vi "Launch.vi"() -> ()   [LabVIEW 2019]
uses:
  Components/ViPER.lvlibp/1abvi3w/ProjectTemplates/Source/Core/ViPER/Components_Src/ViPER/ViPER.lvclass
panel:
  in  "Config XML":string="<?xml version=\"1.0\" encoding=\"UTF-8\" standalone=\"no\" ?>\n<Object>\n\n  <Name>Switch_Mgr</Name>\n\n  <Class>Switch_Manager</Class>\n\n  <Objects>\n    <Object>\n      <Name>Matrix_1</Name>\n      <Class>Switch_Keysight_34934A</Class>\n      <Config>\n        <NumElts>4</NumElts>\n        <Refnum>\n          <Name>VISA</Name>\n          <RefKind>VISA</RefKind>\n          <Val>USB0::0x0957::0x0507::MY56485422::INSTR</Val>\n</Refnum>\n        <I32>\n          <Name>Slot</Name>\n          <Val>1</Val>\n</I32>\n        <Array>\n          <Name>SwitchMap</Name>\n          <Dimsize>65</Dimsize>\n          <Cluster>\n            <Name>Alias</Name>\n            <NumElts>6</NumElts>\n            <String>\n              <Name>Name</Name>\n              <Val>Passive_Tests</Val>\n</String>\n            <Array>\n              <Name>Route</Name>\n              <Dimsize>0</Dimsize>\n              <String>\n                <Name>String</Name>\n                <Val/>\n</String>\n</Array>\n            <Array>\n              <Name>UnRoute</Name>\n              <Dimsize>0</Dimsize>\n              <String>\n                <Name>String</Name>\n                <Val/>\n</String>\n</Array>\n            <String>\n              <Name>Description</Name>\n              <Val>Tests component values unpowered</Val>\n</String>\n            <String>\n              <Name>Group</Name>\n              <Val/>\n</String>\n            <Boolean>\n              <Name>IsGroup</Name>\n              <Val>1</Val>\n</Boolean>\n</Cluster>\n          <Cluster>\n            <Name>Alias</Name>\n            <NumElts>6</NumElts>\n            <String>\n              <Name>Name</Name>\n              <Val>Discharge_C108_C109</Val>\n</String>\n            <Array>\n              <Name>Route</Name>\n              <Dimsize>4</Dimsize>\n              <String>\n                <Name>String</Name>\n                <Val>M1H:1:6:1</Val>\n</String>\n              <String>\n                <Name>String</Name>\n                <Val>M1H:1:19:1</Val>\n</String>\n              <String>\n                <Name>String</Name>\n                <Val>M1L:1:6:1</Val>\n</String>\n              <String>\n                <Name>String</Name>\n                <Val>M1L:1:19:1</Val>\n</String>\n</Array>\n            <Array>\n              <Name>UnRoute</Name>\n              <Dimsize>4</Dimsize>\n              <String>\n                <Name>String</Name>\n                <Val>M1H:1:6:0</Val>\n</String>\n              <String>\n                <Name>String</Name>\n                <Val>M1H:1:19:0</Val>\n</String>\n              <String>\n                <Name>String</Name>\n                <Val>M1L:1:6:0</Val>\n</String>\n              <String>\n                <Name>String</Name>\n                <Val>M1L:1:19:0</Val>\n</String>\n</Array>\n            <String>\n              <Name>Description</Name>\n              <Val>Discharge the caps for 3 secs</Val>\n</String>\n            <String>\n              <Name>Group</Name>\n              <Val>Passive_Tests</Val>\n</String>\n            <Boolean>\n              <Name>IsGroup</Name>\n              <Val>0</Val>\n</Boolean>\n</Cluster>\n          <Cluster>\n            <Name>Alias</Name>\n            <NumElts>6</NumElts>\n            <String>\n              <Name>Name</Name>\n              <Val>Capacitors</Val>\n</String>\n            <Array>\n              <Name>Route</Name>\n              <Dimsize>0</Dimsize>\n              <String>\n                <Name>String</Name>\n                <Val/>\n</String>\n</Array>\n            <Array>\n              <Name>UnRoute</Name>\n              <Dimsize>0</Dimsize>\n              <String>\n                <Name>String</Name>\n                <Val/>\n</String>\n</Array>\n            <String>\n              <Name>Description</Name>\n              <Val>Tests Capacitor Values</Val>\n</String>\n            <String>\n              <Name>Group</Name>\n              <Val>Passive_Tests</Val>\n</String>\n            <Boolean>\n              <Name>IsGroup</Name>\n              <Val>1</Val>\n</Boolean>\n</Cluster>\n          <Cluster>\n            <Name>Alias</Name>\n            <NumElts>6</NumElts>\n            <String>\n              <Name>Name</Name>\n              <Val>Connect_LCR</Val>\n</String>\n            <Array>\n              <Name>Route</Name>\n              <Dimsize>4</Dimsize>\n              <String>\n                <Name>String</Name>\n                <Val>M1H:1:23:1</Val>\n</String>\n              <String>\n                <Name>String</Name>\n                <Val>M1H:2:24:1</Val>\n</String>\n              <String>\n                <Name>String</Name>\n                <Val>M1L:1:25:1</Val>\n</String>\n              <String>\n                <Name>String</Name>\n                <Val>M1L:2:26:1</Val>\n</String>\n</Array>\n            <Array>\n              <Name>UnRoute</Name>\n              <Dimsize>4</Dimsize>\n              <String>\n                <Name>String</Name>\n                <Val>M1H:1:23:0</Val>\n</String>\n              <String>\n                <Name>String</Name>\n                <Val>M1H:2:24:0</Val>\n</String>\n              <String>\n                <Name>String</Name>\n                <Val>M1L:1:25:0</Val>\n</String>\n              <String>\n                <Name>String</Name>\n                <Val>M1L:2:26:0</Val>\n</String>\n</Array>\n            <String>\n              <Name>Description</Name>\n              <Val>Connect the LCR to the Matrix</Val>\n</String>\n            <String>\n              <Name>Group</Name>\n              <Val>Capacitors</Val>\n</String>\n            <Boolean>\n              <Name>IsGroup</Name>\n              <Val>0</Val>\n</Boolean>\n</Cluster>\n          <Cluster>\n            <Name>Alias</Name>\n            <NumElts>6</NumElts>\n            <String>\n              <Name>Name</Name>\n              <Val>C108_C109</Val>\n</String>\n            <Array>\n              <Name>Route</Name>\n              <Dimsize>4</Dimsize>\n              <String>\n                <Name>String</Name>\n                <Val>M1H:1:6:1</Val>\n</String>\n              <String>\n                <Name>String</Name>\n                <Val>M1H:2:6:1</Val>\n</String>\n              <String>\n                <Name>String</Name>\n                <Val>M1L:1:6:1</Val>\n</String>\n              <String>\n                <Name>String</Name>\n                <Val>M1L:2:6:1</Val>\n</String>\n</Array>\n            <Array>\n              <Name>UnRoute</Name>\n              <Dimsize>4</Dimsize>\n              <String>\n                <Name>String</Name>\n                <Val>M1H:1:6:0</Val>\n</String>\n              <String>\n                <Name>String</Name>\n                <Val>M1H:2:6:0</Val>\n</String>\n              <String>\n                <Name>String</Name>\n                <Val>M1L:1:6:0</Val>\n</String>\n              <String>\n                <Name>String</Name>\n                <Val>M1L:2:6:0</Val>\n</String>\n</Array>\n            <String>\n              <Name>Description</Name>\n              <Val>C108 and C109 to LCR</Val>\n</String>\n            <String>\n              <Name>Group</Name>\n              <Val>Capacitors</Val>\n</String>\n            <Boolean>\n              <Name>IsGroup</Name>\n              <Val>0</Val>\n</Boolean>\n</Cluster>\n          <Cluster>\n            <Name>Alias</Name>\n            <NumElts>6</NumElts>\n            <String>\n              <Name>Name</Name>\n              <Val>C153</Val>\n</String>\n            <Array>\n              <Name>Route</Name>\n              <Dimsize>4</Dimsize>\n              <String>\n                <Name>String</Name>\n                <Val>M1H:1:7:1</Val>\n</String>\n              <String>\n                <Name>String</Name>\n                <Val>M1H:2:7:1</Val>\n</String>\n              <String>\n                <Name>String</Name>\n                <Val>M1L:1:5:1</Val>\n</String>\n              <String>\n                <Name>String</Name>\n                <Val>M1L:2:5:1</Val>\n</String>\n</Array>\n            <Array>\n              <Name>UnRoute</Name>\n              <Dimsize>4</Dimsize>\n              <String>\n                <Name>String</Name>\n                <Val>M1H:1:7:0</Val>\n</String>\n              <String>\n                <Name>String</Name>\n                <Val>M1H:2:7:0</Val>\n</String>\n              <String>\n                <Name>String</Name>\n                <Val>M1L:1:5:0</Val>\n</String>\n              <String>\n                <Name>String</Name>\n                <Val>M1L:2:5:0</Val>\n</String>\n</Array>\n            <String>\n              <Name>Description</Name>\n              <Val>C153 to LCR</Val>\n</String>\n            <String>\n              <Name>Group</Name>\n              <Val>Capacitors</Val>\n</String>\n            <Boolean>\n              <Name>IsGroup</Name>\n              <Val>0</Val>\n</Boolean>\n</Cluster>\n          <Cluster>\n            <Name>Alias</Name>\n            <NumElts>6</NumElts>\n            <String>\n              <Name>Name</Name>\n              <Val>C1300</Val>\n</String>\n            <Array>\n              <Name>Route</Name>\n              <Dimsize>4</Dimsize>\n              <String>\n                <Name>String</Name>\n                <Val>M1H:1:2:1</Val>\n</String>\n              <String>\n                <Name>String</Name>\n                <Val>M1H:2:2:1</Val>\n</String>\n              <String>\n                <Name>String</Name>\n                <Val>M1L:1:7:1</Val>\n</String>\n              <String>\n                <Name>String</Name>\n                <Val>M1L:2:7:1</Val>\n</String>\n</Array>\n            <Array>\n              <Name>UnRoute</Name>\n              <Dimsize>4</Dimsize>\n              <String>\n                <Name>String</Name>\n                <Val>M1H:1:2:0</Val>\n</String>\n              <String>\n                <Name>String</Name>\n                <Val>M1H:2:2:0</Val>\n</String>\n              <String>\n                <Name>String</Name>\n                <Val>M1L:1:7:0</Val>\n</String>\n              <String>\n                <Name>String</Name>\n                <Val>M1L:2:7:0</Val>\n</String>\n</Array>\n            <String>\n              <Name>Description</Name>\n              <Val>C1300 to LCR</Val>\n</String>\n            <String>\n              <Name>Group</Name>\n              <Val>Capacitors</Val>\n</String>\n            <Boolean>\n              <Name>IsGroup</Name>\n              <Val>0</Val>\n</Boolean>\n</Cluster>\n          <Cluster>\n            <Name>Alias</Name>\n            <NumElts>6</NumElts>\n            <String>\n              <Name>Name</Name>\n              <Val>C701</Val>\n</String>\n            <Array>\n              <Name>Route</Name>\n              <Dimsize>4</Dimsize>\n              <String>\n                <Name>String</Name>\n                <Val>M1H:1:8:1</Val>\n</String>\n              <String>\n                <Name>String</Name>\n                <Val>M1H:2:8:1</Val>\n</String>\n              <String>\n                <Name>String</Name>\n                <Val>M1L:1:2:1</Val>\n</String>\n              <String>\n                <Name>String</Name>\n                <Val>M1L:2:2:1</Val>\n</String>\n</Array>\n            <Array>\n              <Name>UnRoute</Name>\n              <Dimsize>4</Dimsize>\n              <String>\n                <Name>String</Name>\n                <Val>M1H:1:8:0</Val>\n</String>\n              <String>\n                <Name>String</Name>\n                <Val>M1H:2:8:0</Val>\n</String>\n              <String>\n                <Name>String</Name>\n                <Val>M1L:1:2:0</Val>\n</String>\n              <String>\n                <Name>String</Name>\n                <Val>M1L:2:2:0</Val>\n</String>\n</Array>\n            <String>\n              <Name>Description</Name>\n              <Val>C701 to LCR</Val>\n</String>\n            <String>\n              <Name>Group</Name>\n              <Val>Capacitors</Val>\n</String>\n            <Boolean>\n              <Name>IsGroup</Name>\n              <Val>0</Val>\n</Boolean>\n</Cluster>\n          <Cluster>\n            <Name>Alias</Name>\n            <NumElts>6</NumElts>\n            <String>\n              <Name>Name</Name>\n              <Val>C1202</Val>\n</String>\n            <Array>\n              <Name>Route</Name>\n              <Dimsize>4</Dimsize>\n              <String>\n                <Name>String</Name>\n                <Val>M1H:1:2:1</Val>\n</String>\n              <String>\n                <Name>String</Name>\n                <Val>M1H:2:2:1</Val>\n</String>\n              <String>\n                <Name>String</Name>\n                <Val>M1L:1:8:1</Val>\n</String>\n              <String>\n                <Name>String</Name>\n                <Val>M1L:2:8:1</Val>\n</String>\n</Array>\n            <Array>\n              <Name>UnRoute</Name>\n              <Dimsize>4</Dimsize>\n              <String>\n                <Name>String</Name>\n                <Val>M1H:1:2:0</Val>\n</String>\n              <String>\n                <Name>String</Name>\n                <Val>M1H:2:2:0</Val>\n</String>\n              <String>\n                <Name>String</Name>\n                <Val>M1L:1:8:0</Val>\n</String>\n              <String>\n                <Name>String</Name>\n                <Val>M1L:2:8:0</Val>\n</String>\n</Array>\n            <String>\n              <Name>Description</Name>\n              <Val>C1202 to LCR</Val>\n</String>\n            <String>\n              <Name>Group</Name>\n              <Val>Capacitors</Val>\n</String>\n            <Boolean>\n              <Name>IsGroup</Name>\n              <Val>0</Val>\n</Boolean>\n</Cluster>\n          <Cluster>\n            <Name>Alias</Name>\n            <NumElts>6</NumElts>\n            <String>\n              <Name>Name</Name>\n              <Val>C1204</Val>\n</String>\n            <Array>\n              <Name>Route</Name>\n              <Dimsize>4</Dimsize>\n              <String>\n                <Name>String</Name>\n                <Val>M1H:1:9:1</Val>\n</String>\n              <String>\n                <Name>String</Name>\n                <Val>M1H:2:9:1</Val>\n</String>\n              <String>\n                <Name>String</Name>\n                <Val>M1L:1:2:1</Val>\n</String>\n              <String>\n                <Name>String</Name>\n                <Val>M1L:2:2:1</Val>\n</String>\n</Array>\n            <Array>\n              <Name>UnRoute</Name>\n              <Dimsize>4</Dimsize>\n              <String>\n                <Name>String</Name>\n                <Val>M1H:1:9:0</Val>\n</String>\n              <String>\n                <Name>String</Name>\n                <Val>M1H:2:9:0</Val>\n</String>\n              <String>\n                <Name>String</Name>\n                <Val>M1L:1:2:0</Val>\n</String>\n              <String>\n                <Name>String</Name>\n                <Val>M1L:2:2:0</Val>\n</String>\n</Array>\n            <String>\n              <Name>Description</Name>\n              <Val>C1204 to LCR</Val>\n</String>\n            <String>\n              <Name>Group</Name>\n              <Val>Capacitors</Val>\n</String>\n            <Boolean>\n              <Name>IsGroup</Name>\n              <Val>0</Val>\n</Boolean>\n</Cluster>\n          <Cluster>\n            <Name>Alias</Name>\n            <NumElts>6</NumElts>\n            <String>\n              <Name>Name</Name>\n              <Val>C1200</Val>\n</String>\n            <Array>\n              <Name>Route</Name>\n              <Dimsize>4</Dimsize>\n              <String>\n                <Name>String</Name>\n                <Val>M1H:1:2:1</Val>\n</String>\n              <String>\n                <Name>String</Name>\n                <Val>M1H:2:2:1</Val>\n</String>\n              <String>\n                <Name>String</Name>\n                <Val>M1L:1:9:1</Val>\n</String>\n              <String>\n                <Name>String</Name>\n                <Val>M1L:2:9:1</Val>\n</String>\n</Array>\n            <Array>\n              <Name>UnRoute</Name>\n              <Dimsize>4</Dimsize>\n              <String>\n                <Name>String</Name>\n                <Val>M1H:1:2:0</Val>\n</String>\n              <String>\n                <Name>String</Name>\n                <Val>M1H:2:2:0</Val>\n</String>\n              <String>\n                <Name>String</Name>\n                <Val>M1L:1:9:0</Val>\n</String>\n              <String>\n                <Name>String</Name>\n                <Val>M1L:2:9:0</Val>\n</String>\n</Array>\n            <String>\n              <Name>Description</Name>\n              <Val>C1200 to LCR</Val>\n</String>\n            <String>\n              <Name>Group</Name>\n              <Val>Capacitors</Val>\n</String>\n            <Boolean>\n              <Name>IsGroup</Name>\n              <Val>0</Val>\n</Boolean>\n</Cluster>\n          <Cluster>\n            <Name>Alias</Name>\n            <NumElts>6</NumElts>\n            <String>\n              <Name>Name</Name>\n              <Val>Resistors</Val>\n</String>\n            <Array>\n              <Name>Route</Name>\n              <Dimsize>0</Dimsize>\n              <String>\n                <Name>String</Name>\n                <Val/>\n</String>\n</Array>\n            <Array>\n              <Name>UnRoute</Name>\n              <Dimsize>0</Dimsize>\n              <String>\n                <Name>String</Name>\n                <Val/>\n</String>\n</Array>\n            <String>\n              <Name>Description</Name>\n              <Val>Connect resistances to the DMM</Val>\n</String>\n            <String>\n              <Name>Group</Name>\n              <Val>Passive_Tests</Val>\n</String>\n            <Boolean>\n              <Name>IsGroup</Name>\n              <Val>1</Val>\n</Boolean>\n</Cluster>\n          <Cluster>\n            <Name>Alias</Name>\n            <NumElts>6</NumElts>\n            <String>\n              <Name>Name</Name>\n              <Val>24V_to_Gnd</Val>\n</String>\n            <Array>\n              <Name>Route</Name>\n              <Dimsize>0</Dimsize>\n              <String>\n                <Name>String</Name>\n                <Val/>\n</String>\n</Array>\n            <Array>\n              <Name>UnRoute</Name>\n              <Dimsize>0</Dimsize>\n              <String>\n                <Name>String</Name>\n                <Val/>\n</String>\n</Array>\n            <String>\n              <Name>Description</Name>\n              <Val>Ensure supply is not short circuit</Val>\n</String>\n            <String>\n              <Name>Group</Name>\n              <Val>Resistors</Val>\n</String>\n            <Boolean>\n              <Name>IsGroup</Name>\n              <Val>0</Val>\n</Boolean>\n</Cluster>\n          <Cluster>\n            <Name>Alias</Name>\n            <NumElts>6</NumElts>\n            <String>\n              <Name>Name</Name>\n              <Val>R121</Val>\n</String>\n            <Array>\n              <Name>Route</Name>\n              <Dimsize>4</Dimsize>\n              <String>\n                <Name>String</Name>\n                <Val>M1H:1:3:1</Val>\n</String>\n              <String>\n                <Name>String</Name>\n                <Val>M1H:2:3:1</Val>\n</String>\n              <String>\n                <Name>String</Name>\n                <Val>M1H:3:5:1</Val>\n</String>\n              <String>\n                <Name>String</Name>\n                <Val>M1H:4:5:1</Val>\n</String>\n</Array>\n            <Array>\n              <Name>UnRoute</Name>\n              <Dimsize>4</Dimsize>\n              <String>\n                <Name>String</Name>\n                <Val>M1H:1:3:0</Val>\n</String>\n              <String>\n                <Name>String</Name>\n                <Val>M1H:2:3:0</Val>\n</String>\n              <String>\n                <Name>String</Name>\n                <Val>M1H:3:5:0</Val>\n</String>\n              <String>\n                <Name>String</Name>\n                <Val>M1H:4:5:0</Val>\n</String>\n</Array>\n            <String>\n              <Name>Description</Name>\n              <Val>R121 to DMM</Val>\n</String>\n            <String>\n              <Name>Group</Name>\n              <Val>Resistors</Val>\n</String>\n            <Boolean>\n              <Name>IsGroup</Name>\n              <Val>0</Val>\n</Boolean>\n</Cluster>\n          <Cluster>\n            <Name>Alias</Name>\n            <NumElts>6</NumElts>\n            <String>\n              <Name>Name</Name>\n              <Val>LUG</Val>\n</String>\n            <Array>\n              <Name>Route</Name>\n              <Dimsize>4</Dimsize>\n              <String>\n                <Name>String</Name>\n                <Val>M1H:1:10:1</Val>\n</String>\n              <String>\n                <Name>String</Name>\n                <Val>M1H:2:10:1</Val>\n</String>\n              <String>\n                <Name>String</Name>\n                <Val>M1H:3:2:1</Val>\n</String>\n              <String>\n                <Name>String</Name>\n                <Val>M1H:4:2:1</Val>\n</String>\n</Array>\n            <Array>\n              <Name>UnRoute</Name>\n              <Dimsize>4</Dimsize>\n              <String>\n                <Name>String</Name>\n                <Val>M1H:1:10:0</Val>\n</String>\n              <String>\n                <Name>String</Name>\n                <Val>M1H:2:10:0</Val>\n</String>\n              <String>\n                <Name>String</Name>\n                <Val>M1H:3:2:0</Val>\n</String>\n              <String>\n                <Name>String</Name>\n                <Val>M1H:4:2:0</Val>\n</String>\n</Array>\n            <String>\n              <Name>Description</Name>\n              <Val>LUG to DMM</Val>\n</String>\n            <String>\n              <Name>Group</Name>\n              <Val>Resistors</Val>\n</String>\n            <Boolean>\n              <Name>IsGroup</Name>\n              <Val>0</Val>\n</Boolean>\n</Cluster>\n          <Cluster>\n            <Name>Alias</Name>\n            <NumElts>6</NumElts>\n            <String>\n              <Name>Name</Name>\n              <Val>R304</Val>\n</String>\n            <Array>\n              <Name>Route</Name>\n              <Dimsize>4</Dimsize>\n              <String>\n                <Name>String</Name>\n                <Val>M1L:1:10:1</Val>\n</String>\n              <String>\n                <Name>String</Name>\n                <Val>M1L:2:10:1</Val>\n</String>\n              <String>\n                <Name>String</Name>\n                <Val>M1L:3:2:1</Val>\n</String>\n              <String>\n                <Name>String</Name>\n                <Val>M1L:4:2:1</Val>\n</String>\n</Array>\n            <Array>\n              <Name>UnRoute</Name>\n              <Dimsize>4</Dimsize>\n              <String>\n                <Name>String</Name>\n                <Val>M1L:1:10:0</Val>\n</String>\n              <String>\n                <Name>String</Name>\n                <Val>M1L:2:10:0</Val>\n</String>\n              <String>\n                <Name>String</Name>\n                <Val>M1L:3:2:0</Val>\n</String>\n              <String>\n                <Name>String</Name>\n                <Val>M1L:4:2:0</Val>\n</String>\n</Array>\n            <String>\n              <Name>Description</Name>\n              <Val>R304 to DMM</Val>\n</String>\n            <String>\n              <Name>Group</Name>\n              <Val>Resistors</Val>\n</String>\n            <Boolean>\n              <Name>IsGroup</Name>\n              <Val>0</Val>\n</Boolean>\n</Cluster>\n          <Cluster>\n            <Name>Alias</Name>\n            <NumElts>6</NumElts>\n            <String>\n              <Name>Name</Name>\n              <Val>R203</Val>\n</String>\n            <Array>\n              <Name>Route</Name>\n              <Dimsize>4</Dimsize>\n              <String>\n                <Name>String</Name>\n                <Val>M1H:1:11:1</Val>\n</String>\n              <String>\n                <Name>String</Name>\n                <Val>M1H:2:11:1</Val>\n</String>\n              <String>\n                <Name>String</Name>\n                <Val>M1L:3:11:1</Val>\n</String>\n              <String>\n                <Name>String</Name>\n                <Val>M1L:4:11:1</Val>\n</String>\n</Array>\n            <Array>\n              <Name>UnRoute</Name>\n              <Dimsize>4</Dimsize>\n              <String>\n                <Name>String</Name>\n                <Val>M1H:1:11:0</Val>\n</String>\n              <String>\n                <Name>String</Name>\n                <Val>M1H:2:11:0</Val>\n</String>\n              <String>\n                <Name>String</Name>\n                <Val>M1L:3:11:0</Val>\n</String>\n              <String>\n                <Name>String</Name>\n                <Val>M1L:4:11:0</Val>\n</String>\n</Array>\n            <String>\n              <Name>Description</Name>\n              <Val>R203 to DMM</Val>\n</String>\n            <String>\n              <Name>Group</Name>\n              <Val>Resistors</Val>\n</String>\n            <Boolean>\n              <Name>IsGroup</Name>\n              <Val>0</Val>\n</Boolean>\n</Cluster>\n          <Cluster>\n            <Name>Alias</Name>\n            <NumElts>6</NumElts>\n            <String>\n              <Name>Name</Name>\n              <Val>R207</Val>\n</String>\n            <Array>\n              <Name>Route</Name>\n              <Dimsize>4</Dimsize>\n              <String>\n                <Name>String</Name>\n                <Val>M1H:1:16:1</Val>\n</String>\n              <String>\n                <Name>String</Name>\n                <Val>M1H:2:16:1</Val>\n</String>\n              <String>\n                <Name>String</Name>\n                <Val>M1L:3:15:1</Val>\n</String>\n              <String>\n                <Name>String</Name>\n                <Val>M1L:4:15:1</Val>\n</String>\n</Array>\n            <Array>\n              <Name>UnRoute</Name>\n              <Dimsize>4</Dimsize>\n              <String>\n                <Name>String</Name>\n                <Val>M1H:1:16:0</Val>\n</String>\n              <String>\n                <Name>String</Name>\n                <Val>M1H:2:16:0</Val>\n</String>\n              <String>\n                <Name>String</Name>\n                <Val>M1L:3:15:0</Val>\n</String>\n              <String>\n                <Name>String</Name>\n                <Val>M1L:4:15:0</Val>\n</String>\n</Array>\n            <String>\n              <Name>Description</Name>\n              <Val>R207 to DMM</Val>\n</String>\n            <String>\n              <Name>Group</Name>\n              <Val>Resistors</Val>\n</String>\n            <Boolean>\n              <Name>IsGroup</Name>\n              <Val>0</Val>\n</Boolean>\n</Cluster>\n          <Cluster>\n            <Name>Alias</Name>\n            <NumElts>6</NumElts>\n            <String>\n              <Name>Name</Name>\n              <Val>R200</Val>\n</String>\n            <Array>\n              <Name>Route</Name>\n              <Dimsize>4</Dimsize>\n              <String>\n                <Name>String</Name>\n                <Val>M1H:1:3:1</Val>\n</String>\n              <String>\n                <Name>String</Name>\n                <Val>M1H:2:3:1</Val>\n</String>\n              <String>\n                <Name>String</Name>\n                <Val>M1L:3:16:1</Val>\n</String>\n              <String>\n                <Name>String</Name>\n                <Val>M1L:4:16:1</Val>\n</String>\n</Array>\n            <Array>\n              <Name>UnRoute</Name>\n              <Dimsize>4</Dimsize>\n              <String>\n                <Name>String</Name>\n                <Val>M1H:1:3:0</Val>\n</String>\n              <String>\n                <Name>String</Name>\n                <Val>M1H:2:3:0</Val>\n</String>\n              <String>\n                <Name>String</Name>\n                <Val>M1L:3:16:0</Val>\n</String>\n              <String>\n                <Name>String</Name>\n                <Val>M1L:4:16:0</Val>\n</String>\n</Array>\n            <String>\n              <Name>Description</Name>\n              <Val>R200 to DMM</Val>\n</String>\n            <String>\n              <Name>Group</Name>\n              <Val>Resistors</Val>\n</String>\n            <Boolean>\n              <Name>IsGroup</Name>\n              <Val>0</Val>\n</Boolean>\n</Cluster>\n          <Cluster>\n            <Name>Alias</Name>\n            <NumElts>6</NumElts>\n            <String>\n              <Name>Name</Name>\n              <Val>R201</Val>\n</String>\n            <Array>\n              <Name>Route</Name>\n              <Dimsize>4</Dimsize>\n              <String>\n                <Name>String</Name>\n                <Val>M1H:1:3:1</Val>\n</String>\n              <String>\n                <Name>String</Name>\n                <Val>M1H:2:3:1</Val>\n</String>\n              <String>\n                <Name>String</Name>\n                <Val>M1H:3:17:1</Val>\n</String>\n              <String>\n                <Name>String</Name>\n                <Val>M1H:4:17:1</Val>\n</String>\n</Array>\n            <Array>\n              <Name>UnRoute</Name>\n              <Dimsize>4</Dimsize>\n              <String>\n                <Name>String</Name>\n                <Val>M1H:1:3:0</Val>\n</String>\n              <String>\n                <Name>String</Name>\n                <Val>M1H:2:3:0</Val>\n</String>\n              <String>\n                <Name>String</Name>\n                <Val>M1H:3:17:0</Val>\n</String>\n              <String>\n                <Name>String</Name>\n                <Val>M1H:4:17:0</Val>\n</String>\n</Array>\n            <String>\n              <Name>Description</Name>\n              <Val>R201 to DMM</Val>\n</String>\n            <String>\n              <Name>Group</Name>\n              <Val>Resistors</Val>\n</String>\n            <Boolean>\n              <Name>IsGroup</Name>\n              <Val>0</Val>\n</Boolean>\n</Cluster>\n          <Cluster>\n            <Name>Alias</Name>\n            <NumElts>6</NumElts>\n            <String>\n              <Name>Name</Name>\n              <Val>R215</Val>\n</String>\n            <Array>\n              <Name>Route</Name>\n              <Dimsize>4</Dimsize>\n              <String>\n                <Name>String</Name>\n                <Val>M1L:1:12:1</Val>\n</String>\n              <String>\n                <Name>String</Name>\n                <Val>M1L:2:12:1</Val>\n</String>\n              <String>\n                <Name>String</Name>\n                <Val>M1L:3:2:1</Val>\n</String>\n              <String>\n                <Name>String</Name>\n                <Val>M1L:4:2:1</Val>\n</String>\n</Array>\n            <Array>\n              <Name>UnRoute</Name>\n              <Dimsize>4</Dimsize>\n              <String>\n                <Name>String</Name>\n                <Val>M1L:1:12:0</Val>\n</String>\n              <String>\n                <Name>String</Name>\n                <Val>M1L:2:12:0</Val>\n</String>\n              <String>\n                <Name>String</Name>\n                <Val>M1L:3:2:0</Val>\n</String>\n              <String>\n                <Name>String</Name>\n                <Val>M1L:4:2:0</Val>\n</String>\n</Array>\n            <String>\n              <Name>Description</Name>\n              <Val>R215 to DMM</Val>\n</String>\n            <String>\n              <Name>Group</Name>\n              <Val>Resistors</Val>\n</String>\n            <Boolean>\n              <Name>IsGroup</Name>\n              <Val>0</Val>\n</Boolean>\n</Cluster>\n          <Cluster>\n            <Name>Alias</Name>\n            <NumElts>6</NumElts>\n            <String>\n              <Name>Name</Name>\n              <Val>R214</Val>\n</String>\n            <Array>\n              <Name>Route</Name>\n              <Dimsize>4</Dimsize>\n              <String>\n                <Name>String</Name>\n                <Val>M1H:1:2:1</Val>\n</String>\n              <String>\n                <Name>String</Name>\n                <Val>M1H:2:2:1</Val>\n</String>\n              <String>\n                <Name>String</Name>\n                <Val>M1L:3:12:1</Val>\n</String>\n              <String>\n                <Name>String</Name>\n                <Val>M1L:4:12:1</Val>\n</String>\n</Array>\n            <Array>\n              <Name>UnRoute</Name>\n              <Dimsize>4</Dimsize>\n              <String>\n                <Name>String</Name>\n                <Val>M1H:1:2:0</Val>\n</String>\n              <String>\n                <Name>String</Name>\n                <Val>M1H:2:2:0</Val>\n</String>\n              <String>\n                <Name>String</Name>\n                <Val>M1L:3:12:0</Val>\n</String>\n              <String>\n                <Name>String</Name>\n                <Val>M1L:4:12:0</Val>\n</String>\n</Array>\n            <String>\n              <Name>Description</Name>\n              <Val>R214 to DMM</Val>\n</String>\n            <String>\n              <Name>Group</Name>\n              <Val>Resistors</Val>\n</String>\n            <Boolean>\n              <Name>IsGroup</Name>\n              <Val>0</Val>\n</Boolean>\n</Cluster>\n          <Cluster>\n            <Name>Alias</Name>\n            <NumElts>6</NumElts>\n            <String>\n              <Name>Name</Name>\n              <Val>R412</Val>\n</String>\n            <Array>\n              <Name>Route</Name>\n              <Dimsize>4</Dimsize>\n              <String>\n                <Name>String</Name>\n                <Val>M1L:1:3:1</Val>\n</String>\n              <String>\n                <Name>String</Name>\n                <Val>M1L:2:3:1</Val>\n</String>\n              <String>\n                <Name>String</Name>\n                <Val>M1L:3:17:1</Val>\n</String>\n              <String>\n                <Name>String</Name>\n                <Val>M1L:4:17:1</Val>\n</String>\n</Array>\n            <Array>\n              <Name>UnRoute</Name>\n              <Dimsize>4</Dimsize>\n              <String>\n                <Name>String</Name>\n                <Val>M1L:1:3:0</Val>\n</String>\n              <String>\n                <Name>String</Name>\n                <Val>M1L:2:3:0</Val>\n</String>\n              <String>\n                <Name>String</Name>\n                <Val>M1L:3:17:0</Val>\n</String>\n              <String>\n                <Name>String</Name>\n                <Val>M1L:4:17:0</Val>\n</String>\n</Array>\n            <String>\n              <Name>Description</Name>\n              <Val>R412 to DMM</Val>\n</String>\n            <String>\n              <Name>Group</Name>\n              <Val>Resistors</Val>\n</String>\n            <Boolean>\n              <Name>IsGroup</Name>\n              <Val>0</Val>\n</Boolean>\n</Cluster>\n          <Cluster>\n            <Name>Alias</Name>\n            <NumElts>6</NumElts>\n            <String>\n              <Name>Name</Name>\n              <Val>R413</Val>\n</String>\n            <Array>\n              <Name>Route</Name>\n              <Dimsize>4</Dimsize>\n              <String>\n                <Name>String</Name>\n                <Val>M1H:1:13:1</Val>\n</String>\n              <String>\n                <Name>String</Name>\n                <Val>M1H:2:13:1</Val>\n</String>\n              <String>\n                <Name>String</Name>\n                <Val>M1H:3:2:1</Val>\n</String>\n              <String>\n                <Name>String</Name>\n                <Val>M1H:4:2:1</Val>\n</String>\n</Array>\n            <Array>\n              <Name>UnRoute</Name>\n              <Dimsize>4</Dimsize>\n              <String>\n                <Name>String</Name>\n                <Val>M1H:1:13:0</Val>\n</String>\n              <String>\n                <Name>String</Name>\n                <Val>M1H:2:13:0</Val>\n</String>\n              <String>\n                <Name>String</Name>\n                <Val>M1H:3:2:0</Val>\n</String>\n              <String>\n                <Name>String</Name>\n                <Val>M1H:4:2:0</Val>\n</String>\n</Array>\n            <String>\n              <Name>Description</Name>\n              <Val>R413 to DMM</Val>\n</String>\n            <String>\n              <Name>Group</Name>\n              <Val>Resistors</Val>\n</String>\n            <Boolean>\n              <Name>IsGroup</Name>\n              <Val>0</Val>\n</Boolean>\n</Cluster>\n          <Cluster>\n            <Name>Alias</Name>\n            <NumElts>6</NumElts>\n            <String>\n              <Name>Name</Name>\n              <Val>R416</Val>\n</String>\n            <Array>\n              <Name>Route</Name>\n              <Dimsize>4</Dimsize>\n              <String>\n                <Name>String</Name>\n                <Val>M1L:1:13:1</Val>\n</String>\n              <String>\n                <Name>String</Name>\n                <Val>M1L:2:13:1</Val>\n</String>\n              <String>\n                <Name>String</Name>\n                <Val>M1L:3:2:1</Val>\n</String>\n              <String>\n                <Name>String</Name>\n                <Val>M1L:4:2:1</Val>\n</String>\n</Array>\n            <Array>\n              <Name>UnRoute</Name>\n              <Dimsize>4</Dimsize>\n              <String>\n                <Name>String</Name>\n                <Val>M1L:1:13:0</Val>\n</String>\n              <String>\n                <Name>String</Name>\n                <Val>M1L:2:13:0</Val>\n</String>\n              <String>\n                <Name>String</Name>\n                <Val>M1L:3:2:0</Val>\n</String>\n              <String>\n                <Name>String</Name>\n                <Val>M1L:4:2:0</Val>\n</String>\n</Array>\n            <String>\n              <Name>Description</Name>\n              <Val>R416 to DMM</Val>\n</String>\n            <String>\n              <Name>Group</Name>\n              <Val>Resistors</Val>\n</String>\n            <Boolean>\n              <Name>IsGroup</Name>\n              <Val>0</Val>\n</Boolean>\n</Cluster>\n          <Cluster>\n            <Name>Alias</Name>\n            <NumElts>6</NumElts>\n            <String>\n              <Name>Name</Name>\n              <Val>SP500</Val>\n</String>\n            <Array>\n              <Name>Route</Name>\n              <Dimsize>4</Dimsize>\n              <String>\n                <Name>String</Name>\n                <Val>M1H:1:14:1</Val>\n</String>\n              <String>\n                <Name>String</Name>\n                <Val>M1H:2:14:1</Val>\n</String>\n              <String>\n                <Name>String</Name>\n                <Val>M1H:3:18:1</Val>\n</String>\n              <String>\n                <Name>String</Name>\n                <Val>M1H:4:18:1</Val>\n</String>\n</Array>\n            <Array>\n              <Name>UnRoute</Name>\n              <Dimsize>4</Dimsize>\n              <String>\n                <Name>String</Name>\n                <Val>M1H:1:14:0</Val>\n</String>\n              <String>\n                <Name>String</Name>\n                <Val>M1H:2:14:0</Val>\n</String>\n              <String>\n                <Name>String</Name>\n                <Val>M1H:3:18:0</Val>\n</String>\n              <String>\n                <Name>String</Name>\n                <Val>M1H:4:18:0</Val>\n</String>\n</Array>\n            <String>\n              <Name>Description</Name>\n              <Val>SP500 to DMM</Val>\n</String>\n            <String>\n              <Name>Group</Name>\n              <Val>Resistors</Val>\n</String>\n            <Boolean>\n              <Name>IsGroup</Name>\n              <Val>0</Val>\n</Boolean>\n</Cluster>\n          <Cluster>\n            <Name>Alias</Name>\n            <NumElts>6</NumElts>\n            <String>\n              <Name>Name</Name>\n              <Val>R1204</Val>\n</String>\n            <Array>\n              <Name>Route</Name>\n              <Dimsize>4</Dimsize>\n              <String>\n                <Name>String</Name>\n                <Val>M1L:1:2:1</Val>\n</String>\n              <String>\n                <Name>String</Name>\n                <Val>M1L:2:2:1</Val>\n</String>\n              <String>\n                <Name>String</Name>\n                <Val>M1L:3:14:1</Val>\n</String>\n              <String>\n                <Name>String</Name>\n                <Val>M1L:4:14:1</Val>\n</String>\n</Array>\n            <Array>\n              <Name>UnRoute</Name>\n              <Dimsize>4</Dimsize>\n              <String>\n                <Name>String</Name>\n                <Val>M1L:1:2:0</Val>\n</String>\n              <String>\n                <Name>String</Name>\n                <Val>M1L:2:2:0</Val>\n</String>\n              <String>\n                <Name>String</Name>\n                <Val>M1L:3:14:0</Val>\n</String>\n              <String>\n                <Name>String</Name>\n                <Val>M1L:4:14:0</Val>\n</String>\n</Array>\n            <String>\n              <Name>Description</Name>\n              <Val>R1204 to DMM</Val>\n</String>\n            <String>\n              <Name>Group</Name>\n              <Val>Resistors</Val>\n</String>\n            <Boolean>\n              <Name>IsGroup</Name>\n              <Val>0</Val>\n</Boolean>\n</Cluster>\n          <Cluster>\n            <Name>Alias</Name>\n            <NumElts>6</NumElts>\n            <String>\n              <Name>Name</Name>\n              <Val>R1205_R1206</Val>\n</String>\n            <Array>\n              <Name>Route</Name>\n              <Dimsize>4</Dimsize>\n              <String>\n                <Name>String</Name>\n                <Val>M1H:1:15:1</Val>\n</String>\n              <String>\n                <Name>String</Name>\n                <Val>M1H:2:15:1</Val>\n</String>\n              <String>\n                <Name>String</Name>\n                <Val>M1L:3:18:1</Val>\n</String>\n              <String>\n                <Name>String</Name>\n                <Val>M1L:4:18:1</Val>\n</String>\n</Array>\n            <Array>\n              <Name>UnRoute</Name>\n              <Dimsize>4</Dimsize>\n              <String>\n                <Name>String</Name>\n                <Val>M1H:1:15:0</Val>\n</String>\n              <String>\n                <Name>String</Name>\n                <Val>M1H:2:15:0</Val>\n</String>\n              <String>\n                <Name>String</Name>\n                <Val>M1L:3:18:0</Val>\n</String>\n              <String>\n                <Name>String</Name>\n                <Val>M1L:4:18:0</Val>\n</String>\n</Array>\n            <String>\n              <Name>Description</Name>\n              <Val>R1205 and R1206 to DMM</Val>\n</String>\n            <String>\n              <Name>Group</Name>\n              <Val>Resistors</Val>\n</String>\n            <Boolean>\n              <Name>IsGroup</Name>\n              <Val>0</Val>\n</Boolean>\n</Cluster>\n          <Cluster>\n            <Name>Alias</Name>\n            <NumElts>6</NumElts>\n            <String>\n              <Name>Name</Name>\n              <Val>Diodes</Val>\n</String>\n            <Array>\n              <Name>Route</Name>\n              <Dimsize>0</Dimsize>\n              <String>\n                <Name>String</Name>\n                <Val/>\n</String>\n</Array>\n            <Array>\n              <Name>UnRoute</Name>\n              <Dimsize>0</Dimsize>\n              <String>\n                <Name>String</Name>\n                <Val/>\n</String>\n</Array>\n            <String>\n              <Name>Description</Name>\n              <Val>Connect Diodes to the DMM with PSU</Val>\n</String>\n            <String>\n              <Name>Group</Name>\n              <Val>Passive_Tests</Val>\n</String>\n            <Boolean>\n              <Name>IsGroup</Name>\n              <Val>1</Val>\n</Boolean>\n</Cluster>\n          <Cluster>\n            <Name>Alias</Name>\n            <NumElts>6</NumElts>\n            <String>\n              <Name>Name</Name>\n              <Val>D1200</Val>\n</String>\n            <Array>\n              <Name>Route</Name>\n              <Dimsize>5</Dimsize>\n              <String>\n                <Name>String</Name>\n                <Val>M1H:1:15:1</Val>\n</String>\n              <String>\n                <Name>String</Name>\n                <Val>M1H:3:2:1</Val>\n</String>\n              <String>\n                <Name>String</Name>\n                <Val>M1H:3:28:1</Val>\n</String>\n              <String>\n                <Name>String</Name>\n                <Val>M1L:2:18:1</Val>\n</String>\n              <String>\n                <Name>String</Name>\n                <Val>M1L:2:27:1</Val>\n</String>\n</Array>\n            <Array>\n              <Name>UnRoute</Name>\n              <Dimsize>5</Dimsize>\n              <String>\n                <Name>String</Name>\n                <Val>M1H:1:15:0</Val>\n</String>\n              <String>\n                <Name>String</Name>\n                <Val>M1H:3:2:0</Val>\n</String>\n              <String>\n                <Name>String</Name>\n                <Val>M1H:3:28:0</Val>\n</String>\n              <String>\n                <Name>String</Name>\n                <Val>M1L:2:18:0</Val>\n</String>\n              <String>\n                <Name>String</Name>\n                <Val>M1L:2:27:0</Val>\n</String>\n</Array>\n            <String>\n              <Name>Description</Name>\n              <Val>D1200 to DMM and PSU</Val>\n</String>\n            <String>\n              <Name>Group</Name>\n              <Val>Diodes</Val>\n</String>\n            <Boolean>\n              <Name>IsGroup</Name>\n              <Val>0</Val>\n</Boolean>\n</Cluster>\n          <Cluster>\n            <Name>Alias</Name>\n            <NumElts>6</NumElts>\n            <String>\n              <Name>Name</Name>\n              <Val>Active_Tests</Val>\n</String>\n            <Array>\n              <Name>Route</Name>\n              <Dimsize>0</Dimsize>\n              <String>\n                <Name>String</Name>\n                <Val/>\n</String>\n</Array>\n            <Array>\n              <Name>UnRoute</Name>\n              <Dimsize>0</Dimsize>\n              <String>\n                <Name>String</Name>\n                <Val/>\n</String>\n</Array>\n            <String>\n              <Name>Description</Name>\n              <Val>Tests under power</Val>\n</String>\n            <String>\n              <Name>Group</Name>\n              <Val/>\n</String>\n            <Boolean>\n              <Name>IsGroup</Name>\n              <Val>1</Val>\n</Boolean>\n</Cluster>\n          <Cluster>\n            <Name>Alias</Name>\n            <NumElts>6</NumElts>\n            <String>\n              <Name>Name</Name>\n              <Val>Voltages</Val>\n</String>\n            <Array>\n              <Name>Route</Name>\n              <Dimsize>0</Dimsize>\n              <String>\n                <Name>String</Name>\n                <Val/>\n</String>\n</Array>\n            <Array>\n              <Name>UnRoute</Name>\n              <Dimsize>0</Dimsize>\n              <String>\n                <Name>String</Name>\n                <Val/>\n</String>\n</Array>\n            <String>\n              <Name>Description</Name>\n              <Val>Connect test points to DMM</Val>\n</String>\n            <String>\n              <Name>Group</Name>\n              <Val>Active_Tests</Val>\n</String>\n            <Boolean>\n              <Name>IsGroup</Name>\n              <Val>1</Val>\n</Boolean>\n</Cluster>\n          <Cluster>\n            <Name>Alias</Name>\n            <NumElts>6</NumElts>\n            <String>\n              <Name>Name</Name>\n              <Val>CON_24VIN</Val>\n</String>\n            <Array>\n              <Name>Route</Name>\n              <Dimsize>2</Dimsize>\n              <String>\n                <Name>String</Name>\n                <Val>M2H:1:2:1</Val>\n</String>\n              <String>\n                <Name>String</Name>\n                <Val>M2L:3:2:1</Val>\n</String>\n</Array>\n            <Array>\n              <Name>UnRoute</Name>\n              <Dimsize>2</Dimsize>\n              <String>\n                <Name>String</Name>\n                <Val>M2H:1:2:0</Val>\n</String>\n              <String>\n                <Name>String</Name>\n                <Val>M2L:3:2:0</Val>\n</String>\n</Array>\n            <String>\n              <Name>Description</Name>\n              <Val>24V line to DMM</Val>\n</String>\n            <String>\n              <Name>Group</Name>\n              <Val>Voltages</Val>\n</String>\n            <Boolean>\n              <Name>IsGroup</Name>\n              <Val>0</Val>\n</Boolean>\n</Cluster>\n          <Cluster>\n            <Name>Alias</Name>\n            <NumElts>6</NumElts>\n            <String>\n              <Name>Name</Name>\n              <Val>CON_Power_Switch</Val>\n</String>\n            <Array>\n              <Name>Route</Name>\n              <Dimsize>2</Dimsize>\n              <String>\n                <Name>String</Name>\n                <Val>M1H:1:6:1</Val>\n</String>\n              <String>\n                <Name>String</Name>\n                <Val>M1L:3:6:1</Val>\n</String>\n</Array>\n            <Array>\n              <Name>UnRoute</Name>\n              <Dimsize>2</Dimsize>\n              <String>\n                <Name>String</Name>\n                <Val>M1H:1:6:0</Val>\n</String>\n              <String>\n                <Name>String</Name>\n                <Val>M1L:3:6:0</Val>\n</String>\n</Array>\n            <String>\n              <Name>Description</Name>\n              <Val>Power Switch to DMM</Val>\n</String>\n            <String>\n              <Name>Group</Name>\n              <Val>Voltages</Val>\n</String>\n            <Boolean>\n              <Name>IsGroup</Name>\n              <Val>0</Val>\n</Boolean>\n</Cluster>\n          <Cluster>\n            <Name>Alias</Name>\n            <NumElts>6</NumElts>\n            <String>\n              <Name>Name</Name>\n              <Val>PSU_24V</Val>\n</String>\n            <Array>\n              <Name>Route</Name>\n              <Dimsize>2</Dimsize>\n              <String>\n                <Name>String</Name>\n                <Val>M2H:1:3:1</Val>\n</String>\n              <String>\n                <Name>String</Name>\n                <Val>M2H:3:1:1</Val>\n</String>\n</Array>\n            <Array>\n              <Name>UnRoute</Name>\n              <Dimsize>2</Dimsize>\n              <String>\n                <Name>String</Name>\n                <Val>M2H:1:3:0</Val>\n</String>\n              <String>\n                <Name>String</Name>\n                <Val>M2H:3:1:0</Val>\n</String>\n</Array>\n            <String>\n              <Name>Description</Name>\n              <Val>PSU 12V to DMM</Val>\n</String>\n            <String>\n              <Name>Group</Name>\n              <Val>Voltages</Val>\n</String>\n            <Boolean>\n              <Name>IsGroup</Name>\n              <Val>0</Val>\n</Boolean>\n</Cluster>\n          <Cluster>\n            <Name>Alias</Name>\n            <NumElts>6</NumElts>\n            <String>\n              <Name>Name</Name>\n              <Val>PSU_5V</Val>\n</String>\n            <Array>\n              <Name>Route</Name>\n              <Dimsize>2</Dimsize>\n              <String>\n                <Name>String</Name>\n                <Val>M2H:1:4:1</Val>\n</String>\n              <String>\n                <Name>String</Name>\n                <Val>M2H:3:1:1</Val>\n</String>\n</Array>\n            <Array>\n              <Name>UnRoute</Name>\n              <Dimsize>2</Dimsize>\n              <String>\n                <Name>String</Name>\n                <Val>M2H:1:4:0</Val>\n</String>\n              <String>\n                <Name>String</Name>\n                <Val>M2H:3:1:0</Val>\n</String>\n</Array>\n            <String>\n              <Name>Description</Name>\n              <Val>PSU 5V to DMM</Val>\n</String>\n            <String>\n              <Name>Group</Name>\n              <Val>Voltages</Val>\n</String>\n            <Boolean>\n              <Name>IsGroup</Name>\n              <Val>0</Val>\n</Boolean>\n</Cluster>\n          <Cluster>\n            <Name>Alias</Name>\n            <NumElts>6</NumElts>\n            <String>\n              <Name>Name</Name>\n              <Val>PSU_3V3</Val>\n</String>\n            <Array>\n              <Name>Route</Name>\n              <Dimsize>2</Dimsize>\n              <String>\n                <Name>String</Name>\n                <Val>M2L:1:4:1</Val>\n</String>\n              <String>\n                <Name>String</Name>\n                <Val>M2H:3:1:1</Val>\n</String>\n</Array>\n            <Array>\n              <Name>UnRoute</Name>\n              <Dimsize>2</Dimsize>\n              <String>\n                <Name>String</Name>\n                <Val>M2L:1:4:0</Val>\n</String>\n              <String>\n                <Name>String</Name>\n                <Val>M2H:3:1:0</Val>\n</String>\n</Array>\n            <String>\n              <Name>Description</Name>\n              <Val>PSU 3V3 to DMM</Val>\n</String>\n            <String>\n              <Name>Group</Name>\n              <Val>Voltages</Val>\n</String>\n            <Boolean>\n              <Name>IsGroup</Name>\n              <Val>0</Val>\n</Boolean>\n</Cluster>\n          <Cluster>\n            <Name>Alias</Name>\n            <NumElts>6</NumElts>\n            <String>\n              <Name>Name</Name>\n              <Val>PSU_AREF_2V5</Val>\n</String>\n            <Array>\n              <Name>Route</Name>\n              <Dimsize>2</Dimsize>\n              <String>\n                <Name>String</Name>\n                <Val>M2H:1:5:1</Val>\n</String>\n              <String>\n                <Name>String</Name>\n                <Val>M2H:3:1:1</Val>\n</String>\n</Array>\n            <Array>\n              <Name>UnRoute</Name>\n              <Dimsize>2</Dimsize>\n              <String>\n                <Name>String</Name>\n                <Val>M2H:1:5:0</Val>\n</String>\n              <String>\n                <Name>String</Name>\n                <Val>M2H:3:1:0</Val>\n</String>\n</Array>\n            <String>\n              <Name>Description</Name>\n              <Val>PSU AREF 2V5 to DMM</Val>\n</String>\n            <String>\n              <Name>Group</Name>\n              <Val>Voltages</Val>\n</String>\n            <Boolean>\n              <Name>IsGroup</Name>\n              <Val>0</Val>\n</Boolean>\n</Cluster>\n          <Cluster>\n            <Name>Alias</Name>\n            <NumElts>6</NumElts>\n            <String>\n              <Name>Name</Name>\n              <Val>PSU_AREF_1V25</Val>\n</String>\n            <Array>\n              <Name>Route</Name>\n              <Dimsize>2</Dimsize>\n              <String>\n                <Name>String</Name>\n                <Val>M2L:1:5:1</Val>\n</String>\n              <String>\n                <Name>String</Name>\n                <Val>M2H:3:1:1</Val>\n</String>\n</Array>\n            <Array>\n              <Name>UnRoute</Name>\n              <Dimsize>2</Dimsize>\n              <String>\n                <Name>String</Name>\n                <Val>M2L:1:5:0</Val>\n</String>\n              <String>\n                <Name>String</Name>\n                <Val>M2H:3:1:0</Val>\n</String>\n</Array>\n            <String>\n              <Name>Description</Name>\n              <Val>PSU AREF 1V25 to DMM</Val>\n</String>\n            <String>\n              <Name>Group</Name>\n              <Val>Voltages</Val>\n</String>\n            <Boolean>\n              <Name>IsGroup</Name>\n              <Val>0</Val>\n</Boolean>\n</Cluster>\n          <Cluster>\n            <Name>Alias</Name>\n            <NumElts>6</NumElts>\n            <String>\n              <Name>Name</Name>\n              <Val>PSU_4V8</Val>\n</String>\n            <Array>\n              <Name>Route</Name>\n              <Dimsize>2</Dimsize>\n              <String>\n                <Name>String</Name>\n                <Val>M2H:1:6:1</Val>\n</String>\n              <String>\n                <Name>String</Name>\n                <Val>M2H:3:1:1</Val>\n</String>\n</Array>\n            <Array>\n              <Name>UnRoute</Name>\n              <Dimsize>2</Dimsize>\n              <String>\n                <Name>String</Name>\n                <Val>M2H:1:6:0</Val>\n</String>\n              <String>\n                <Name>String</Name>\n                <Val>M2H:3:1:0</Val>\n</String>\n</Array>\n            <String>\n              <Name>Description</Name>\n              <Val>PSU 4V8to DMM</Val>\n</String>\n            <String>\n              <Name>Group</Name>\n              <Val>Voltages</Val>\n</String>\n            <Boolean>\n              <Name>IsGroup</Name>\n              <Val>0</Val>\n</Boolean>\n</Cluster>\n          <Cluster>\n            <Name>Alias</Name>\n            <NumElts>6</NumElts>\n            <String>\n              <Name>Name</Name>\n              <Val>PSU_PWR_GOOD</Val>\n</String>\n            <Array>\n              <Name>Route</Name>\n              <Dimsize>5</Dimsize>\n              <String>\n                <Name>String</Name>\n                <Val>M2H:1:6:1</Val>\n</String>\n              <String>\n                <Name>String</Name>\n                <Val>M2H:1:27:1</Val>\n</String>\n              <String>\n                <Name>String</Name>\n                <Val>M2H:3:28:1</Val>\n</String>\n              <String>\n                <Name>String</Name>\n                <Val>M2L:1:6:1</Val>\n</String>\n              <String>\n                <Name>String</Name>\n                <Val>M2H:3:1:1</Val>\n</String>\n</Array>\n            <Array>\n              <Name>UnRoute</Name>\n              <Dimsize>5</Dimsize>\n              <String>\n                <Name>String</Name>\n                <Val>M2H:1:6:0</Val>\n</String>\n              <String>\n                <Name>String</Name>\n                <Val>M2H:1:27:0</Val>\n</String>\n              <String>\n                <Name>String</Name>\n                <Val>M2H:3:28:0</Val>\n</String>\n              <String>\n                <Name>String</Name>\n                <Val>M2L:1:6:0</Val>\n</String>\n              <String>\n                <Name>String</Name>\n                <Val>M2H:3:1:0</Val>\n</String>\n</Array>\n            <String>\n              <Name>Description</Name>\n              <Val>Connects PWR GOOD to PSU and DMM</Val>\n</String>\n            <String>\n              <Name>Group</Name>\n              <Val>Voltages</Val>\n</String>\n            <Boolean>\n              <Name>IsGroup</Name>\n              <Val>0</Val>\n</Boolean>\n</Cluster>\n          <Cluster>\n            <Name>Alias</Name>\n            <NumElts>6</NumElts>\n            <String>\n              <Name>Name</Name>\n              <Val>PSU_3V3_ANA</Val>\n</String>\n            <Array>\n              <Name>Route</Name>\n              <Dimsize>2</Dimsize>\n              <String>\n                <Name>String</Name>\n                <Val>M2H:1:7:1</Val>\n</String>\n              <String>\n                <Name>String</Name>\n                <Val>M2H:3:1:1</Val>\n</String>\n</Array>\n            <Array>\n              <Name>UnRoute</Name>\n              <Dimsize>2</Dimsize>\n              <String>\n                <Name>String</Name>\n                <Val>M2H:1:7:0</Val>\n</String>\n              <String>\n                <Name>String</Name>\n                <Val>M2H:3:1:0</Val>\n</String>\n</Array>\n            <String>\n              <Name>Description</Name>\n              <Val>Connects PSU 3V3 ANA to DMM</Val>\n</String>\n            <String>\n              <Name>Group</Name>\n              <Val>Voltages</Val>\n</String>\n            <Boolean>\n              <Name>IsGroup</Name>\n              <Val>0</Val>\n</Boolean>\n</Cluster>\n          <Cluster>\n            <Name>Alias</Name>\n            <NumElts>6</NumElts>\n            <String>\n              <Name>Name</Name>\n              <Val>PSU_WDOG_STAT</Val>\n</String>\n            <Array>\n              <Name>Route</Name>\n              <Dimsize>2</Dimsize>\n              <String>\n                <Name>String</Name>\n                <Val>M2H:1:7:1</Val>\n</String>\n              <String>\n                <Name>String</Name>\n                <Val>M2H:3:1:1</Val>\n</String>\n</Array>\n            <Array>\n              <Name>UnRoute</Name>\n              <Dimsize>2</Dimsize>\n              <String>\n                <Name>String</Name>\n                <Val>M2H:1:7:0</Val>\n</String>\n              <String>\n                <Name>String</Name>\n                <Val>M2H:3:1:0</Val>\n</String>\n</Array>\n            <String>\n              <Name>Description</Name>\n              <Val>Connects PSU WDOG STAT to DMM</Val>\n</String>\n            <String>\n              <Name>Group</Name>\n              <Val>Voltages</Val>\n</String>\n            <Boolean>\n              <Name>IsGroup</Name>\n              <Val>0</Val>\n</Boolean>\n</Cluster>\n          <Cluster>\n            <Name>Alias</Name>\n            <NumElts>6</NumElts>\n            <String>\n              <Name>Name</Name>\n              <Val>PSU_WDOG_24V</Val>\n</String>\n            <Array>\n              <Name>Route</Name>\n              <Dimsize>2</Dimsize>\n              <String>\n                <Name>String</Name>\n                <Val>M2H:1:8:1</Val>\n</String>\n              <String>\n                <Name>String</Name>\n                <Val>M2H:3:1:1</Val>\n</String>\n</Array>\n            <Array>\n              <Name>UnRoute</Name>\n              <Dimsize>2</Dimsize>\n              <String>\n                <Name>String</Name>\n                <Val>M2H:1:8:0</Val>\n</String>\n              <String>\n                <Name>String</Name>\n                <Val>M2H:3:1:0</Val>\n</String>\n</Array>\n            <String>\n              <Name>Description</Name>\n              <Val>Connects PSU WDOG 24V to DMM</Val>\n</String>\n            <String>\n              <Name>Group</Name>\n              <Val>Voltages</Val>\n</String>\n            <Boolean>\n              <Name>IsGroup</Name>\n              <Val>0</Val>\n</Boolean>\n</Cluster>\n          <Cluster>\n            <Name>Alias</Name>\n            <NumElts>6</NumElts>\n            <String>\n              <Name>Name</Name>\n              <Val>Valve1</Val>\n</String>\n            <Array>\n              <Name>Route</Name>\n              <Dimsize>2</Dimsize>\n              <String>\n                <Name>String</Name>\n                <Val>M2H:3:9:1</Val>\n</String>\n              <String>\n                <Name>String</Name>\n                <Val>M2H:1:8:1</Val>\n</String>\n</Array>\n            <Array>\n              <Name>UnRoute</Name>\n              <Dimsize>2</Dimsize>\n              <String>\n                <Name>String</Name>\n                <Val>M2H:3:9:0</Val>\n</String>\n              <String>\n                <Name>String</Name>\n                <Val>M2H:1:8:0</Val>\n</String>\n</Array>\n            <String>\n              <Name>Description</Name>\n              <Val>Valve1 to DMM</Val>\n</String>\n            <String>\n              <Name>Group</Name>\n              <Val>Voltages</Val>\n</String>\n            <Boolean>\n              <Name>IsGroup</Name>\n              <Val>0</Val>\n</Boolean>\n</Cluster>\n          <Cluster>\n            <Name>Alias</Name>\n            <NumElts>6</NumElts>\n            <String>\n              <Name>Name</Name>\n              <Val>Valve2</Val>\n</String>\n            <Array>\n              <Name>Route</Name>\n              <Dimsize>2</Dimsize>\n              <String>\n                <Name>String</Name>\n                <Val>M2L:3:9:1</Val>\n</String>\n              <String>\n                <Name>String</Name>\n                <Val>M2H:1:8:1</Val>\n</String>\n</Array>\n            <Array>\n              <Name>UnRoute</Name>\n              <Dimsize>2</Dimsize>\n              <String>\n                <Name>String</Name>\n                <Val>M2L:3:9:0</Val>\n</String>\n              <String>\n                <Name>String</Name>\n                <Val>M2H:1:8:0</Val>\n</String>\n</Array>\n            <String>\n              <Name>Description</Name>\n              <Val>Valve2 to DMM</Val>\n</String>\n            <String>\n              <Name>Group</Name>\n              <Val>Voltages</Val>\n</String>\n            <Boolean>\n              <Name>IsGroup</Name>\n              <Val>0</Val>\n</Boolean>\n</Cluster>\n          <Cluster>\n            <Name>Alias</Name>\n            <NumElts>6</NumElts>\n            <String>\n              <Name>Name</Name>\n              <Val>Valve3</Val>\n</String>\n            <Array>\n              <Name>Route</Name>\n              <Dimsize>2</Dimsize>\n              <String>\n                <Name>String</Name>\n                <Val>M2H:3:10:1</Val>\n</String>\n              <String>\n                <Name>String</Name>\n                <Val>M2H:1:8:1</Val>\n</String>\n</Array>\n            <Array>\n              <Name>UnRoute</Name>\n              <Dimsize>2</Dimsize>\n              <String>\n                <Name>String</Name>\n                <Val>M2H:3:10:0</Val>\n</String>\n              <String>\n                <Name>String</Name>\n                <Val>M2H:1:8:0</Val>\n</String>\n</Array>\n            <String>\n              <Name>Description</Name>\n              <Val>Valve3 to DMM</Val>\n</String>\n            <String>\n              <Name>Group</Name>\n              <Val>Voltages</Val>\n</String>\n            <Boolean>\n              <Name>IsGroup</Name>\n              <Val>0</Val>\n</Boolean>\n</Cluster>\n          <Cluster>\n            <Name>Alias</Name>\n            <NumElts>6</NumElts>\n            <String>\n              <Name>Name</Name>\n              <Val>Valve4</Val>\n</String>\n            <Array>\n              <Name>Route</Name>\n              <Dimsize>2</Dimsize>\n              <String>\n                <Name>String</Name>\n                <Val>M2H:3:11:1</Val>\n</String>\n              <String>\n                <Name>String</Name>\n                <Val>M2H:1:8:1</Val>\n</String>\n</Array>\n            <Array>\n              <Name>UnRoute</Name>\n              <Dimsize>2</Dimsize>\n              <String>\n                <Name>String</Name>\n                <Val>M2H:3:11:0</Val>\n</String>\n              <String>\n                <Name>String</Name>\n                <Val>M2H:1:8:0</Val>\n</String>\n</Array>\n            <String>\n              <Name>Description</Name>\n              <Val>Valve4 to DMM</Val>\n</String>\n            <String>\n              <Name>Group</Name>\n              <Val>Voltages</Val>\n</String>\n            <Boolean>\n              <Name>IsGroup</Name>\n              <Val>0</Val>\n</Boolean>\n</Cluster>\n          <Cluster>\n            <Name>Alias</Name>\n            <NumElts>6</NumElts>\n            <String>\n              <Name>Name</Name>\n              <Val>Valve5</Val>\n</String>\n            <Array>\n              <Name>Route</Name>\n              <Dimsize>2</Dimsize>\n              <String>\n                <Name>String</Name>\n                <Val>M2H:3:11:1</Val>\n</String>\n              <String>\n                <Name>String</Name>\n                <Val>M2H:1:8:1</Val>\n</String>\n</Array>\n            <Array>\n              <Name>UnRoute</Name>\n              <Dimsize>2</Dimsize>\n              <String>\n                <Name>String</Name>\n                <Val>M2H:3:11:0</Val>\n</String>\n              <String>\n                <Name>String</Name>\n                <Val>M2H:1:8:0</Val>\n</String>\n</Array>\n            <String>\n              <Name>Description</Name>\n              <Val>Valve5 to DMM</Val>\n</String>\n            <String>\n              <Name>Group</Name>\n              <Val>Voltages</Val>\n</String>\n            <Boolean>\n              <Name>IsGroup</Name>\n              <Val>0</Val>\n</Boolean>\n</Cluster>\n          <Cluster>\n            <Name>Alias</Name>\n            <NumElts>6</NumElts>\n            <String>\n              <Name>Name</Name>\n              <Val>Valve6</Val>\n</String>\n            <Array>\n              <Name>Route</Name>\n              <Dimsize>2</Dimsize>\n              <String>\n                <Name>String</Name>\n                <Val>M2L:3:11:1</Val>\n</String>\n              <String>\n                <Name>String</Name>\n                <Val>M2H:1:8:1</Val>\n</String>\n</Array>\n            <Array>\n              <Name>UnRoute</Name>\n              <Dimsize>2</Dimsize>\n              <String>\n                <Name>String</Name>\n                <Val>M2L:3:11:0</Val>\n</String>\n              <String>\n                <Name>String</Name>\n                <Val>M2H:1:8:0</Val>\n</String>\n</Array>\n            <String>\n              <Name>Description</Name>\n              <Val>Valve6 to DMM</Val>\n</String>\n            <String>\n              <Name>Group</Name>\n              <Val>Voltages</Val>\n</String>\n            <Boolean>\n              <Name>IsGroup</Name>\n              <Val>0</Val>\n</Boolean>\n</Cluster>\n          <Cluster>\n            <Name>Alias</Name>\n            <NumElts>6</NumElts>\n            <String>\n              <Name>Name</Name>\n              <Val>Valve7</Val>\n</String>\n            <Array>\n              <Name>Route</Name>\n              <Dimsize>2</Dimsize>\n              <String>\n                <Name>String</Name>\n                <Val>M2H:3:12:1</Val>\n</String>\n              <String>\n                <Name>String</Name>\n                <Val>M2H:1:8:1</Val>\n</String>\n</Array>\n            <Array>\n              <Name>UnRoute</Name>\n              <Dimsize>2</Dimsize>\n              <String>\n                <Name>String</Name>\n                <Val>M2H:3:12:0</Val>\n</String>\n              <String>\n                <Name>String</Name>\n                <Val>M2H:1:8:0</Val>\n</String>\n</Array>\n            <String>\n              <Name>Description</Name>\n              <Val>Valve7 to DMM</Val>\n</String>\n            <String>\n              <Name>Group</Name>\n              <Val>Voltages</Val>\n</String>\n            <Boolean>\n              <Name>IsGroup</Name>\n              <Val>0</Val>\n</Boolean>\n</Cluster>\n          <Cluster>\n            <Name>Alias</Name>\n            <NumElts>6</NumElts>\n            <String>\n              <Name>Name</Name>\n              <Val>Valve8</Val>\n</String>\n            <Array>\n              <Name>Route</Name>\n              <Dimsize>2</Dimsize>\n              <String>\n                <Name>String</Name>\n                <Val>M2L:3:12:1</Val>\n</String>\n              <String>\n                <Name>String</Name>\n                <Val>M2H:1:8:1</Val>\n</String>\n</Array>\n            <Array>\n              <Name>UnRoute</Name>\n              <Dimsize>2</Dimsize>\n              <String>\n                <Name>String</Name>\n                <Val>M2L:3:12:0</Val>\n</String>\n              <String>\n                <Name>String</Name>\n                <Val>M2H:1:8:0</Val>\n</String>\n</Array>\n            <String>\n              <Name>Description</Name>\n              <Val>Valve8 to DMM</Val>\n</String>\n            <String>\n              <Name>Group</Name>\n              <Val>Voltages</Val>\n</String>\n            <Boolean>\n              <Name>IsGroup</Name>\n              <Val>0</Val>\n</Boolean>\n</Cluster>\n          <Cluster>\n            <Name>Alias</Name>\n            <NumElts>6</NumElts>\n            <String>\n              <Name>Name</Name>\n              <Val>ValveDrain</Val>\n</String>\n            <Array>\n              <Name>Route</Name>\n              <Dimsize>2</Dimsize>\n              <String>\n                <Name>String</Name>\n                <Val>M2L:3:12:1</Val>\n</String>\n              <String>\n                <Name>String</Name>\n                <Val>M2H:1:8:1</Val>\n</String>\n</Array>\n            <Array>\n              <Name>UnRoute</Name>\n              <Dimsize>2</Dimsize>\n              <String>\n                <Name>String</Name>\n                <Val>M2L:3:12:0</Val>\n</String>\n              <String>\n                <Name>String</Name>\n                <Val>M2H:1:8:0</Val>\n</String>\n</Array>\n            <String>\n              <Name>Description</Name>\n              <Val>ValveDrain to DMM</Val>\n</String>\n            <String>\n              <Name>Group</Name>\n              <Val>Voltages</Val>\n</String>\n            <Boolean>\n              <Name>IsGroup</Name>\n              <Val>0</Val>\n</Boolean>\n</Cluster>\n          <Cluster>\n            <Name>Alias</Name>\n            <NumElts>6</NumElts>\n            <String>\n              <Name>Name</Name>\n              <Val>ValveTemp</Val>\n</String>\n            <Array>\n              <Name>Route</Name>\n              <Dimsize>2</Dimsize>\n              <String>\n                <Name>String</Name>\n                <Val>M2L:3:13:1</Val>\n</String>\n              <String>\n                <Name>String</Name>\n                <Val>M2H:1:8:1</Val>\n</String>\n</Array>\n            <Array>\n              <Name>UnRoute</Name>\n              <Dimsize>2</Dimsize>\n              <String>\n                <Name>String</Name>\n                <Val>M2L:3:13:0</Val>\n</String>\n              <String>\n                <Name>String</Name>\n                <Val>M2H:1:8:0</Val>\n</String>\n</Array>\n            <String>\n              <Name>Description</Name>\n              <Val>ValveTemp to DMM</Val>\n</String>\n            <String>\n              <Name>Group</Name>\n              <Val>Voltages</Val>\n</String>\n            <Boolean>\n              <Name>IsGroup</Name>\n              <Val>0</Val>\n</Boolean>\n</Cluster>\n          <Cluster>\n            <Name>Alias</Name>\n            <NumElts>6</NumElts>\n            <String>\n              <Name>Name</Name>\n              <Val>ValvePump</Val>\n</String>\n            <Array>\n              <Name>Route</Name>\n              <Dimsize>2</Dimsize>\n              <String>\n                <Name>String</Name>\n                <Val>M2H:3:14:1</Val>\n</String>\n              <String>\n                <Name>String</Name>\n                <Val>M2H:1:8:1</Val>\n</String>\n</Array>\n            <Array>\n              <Name>UnRoute</Name>\n              <Dimsize>2</Dimsize>\n              <String>\n                <Name>String</Name>\n                <Val>M2H:3:14:0</Val>\n</String>\n              <String>\n                <Name>String</Name>\n                <Val>M2H:1:8:0</Val>\n</String>\n</Array>\n            <String>\n              <Name>Description</Name>\n              <Val>ValvePump to DMM</Val>\n</String>\n            <String>\n              <Name>Group</Name>\n              <Val>Voltages</Val>\n</String>\n            <Boolean>\n              <Name>IsGroup</Name>\n              <Val>0</Val>\n</Boolean>\n</Cluster>\n          <Cluster>\n            <Name>Alias</Name>\n            <NumElts>6</NumElts>\n            <String>\n              <Name>Name</Name>\n              <Val>ValveLarge</Val>\n</String>\n            <Array>\n              <Name>Route</Name>\n              <Dimsize>2</Dimsize>\n              <String>\n                <Name>String</Name>\n                <Val>M2H:3:14:1</Val>\n</String>\n              <String>\n                <Name>String</Name>\n                <Val>M2H:1:8:1</Val>\n</String>\n</Array>\n            <Array>\n              <Name>UnRoute</Name>\n              <Dimsize>2</Dimsize>\n              <String>\n                <Name>String</Name>\n                <Val>M2H:3:14:0</Val>\n</String>\n              <String>\n                <Name>String</Name>\n                <Val>M2H:1:8:0</Val>\n</String>\n</Array>\n            <String>\n              <Name>Description</Name>\n              <Val>ValveLarge to DMM</Val>\n</String>\n            <String>\n              <Name>Group</Name>\n              <Val>Voltages</Val>\n</String>\n            <Boolean>\n              <Name>IsGroup</Name>\n              <Val>0</Val>\n</Boolean>\n</Cluster>\n          <Cluster>\n            <Name>Alias</Name>\n            <NumElts>6</NumElts>\n            <String>\n              <Name>Name</Name>\n              <Val>ValveSmall</Val>\n</String>\n            <Array>\n              <Name>Route</Name>\n              <Dimsize>2</Dimsize>\n              <String>\n                <Name>String</Name>\n                <Val>M2H:3:14:1</Val>\n</String>\n              <String>\n                <Name>String</Name>\n                <Val>M2H:1:8:1</Val>\n</String>\n</Array>\n            <Array>\n              <Name>UnRoute</Name>\n              <Dimsize>2</Dimsize>\n              <String>\n                <Name>String</Name>\n                <Val>M2H:3:14:0</Val>\n</String>\n              <String>\n                <Name>String</Name>\n                <Val>M2H:1:8:0</Val>\n</String>\n</Array>\n            <String>\n              <Name>Description</Name>\n              <Val>ValveSmall to DMM</Val>\n</String>\n            <String>\n              <Name>Group</Name>\n              <Val>Voltages</Val>\n</String>\n            <Boolean>\n              <Name>IsGroup</Name>\n              <Val>0</Val>\n</Boolean>\n</Cluster>\n          <Cluster>\n            <Name>Alias</Name>\n            <NumElts>6</NumElts>\n            <String>\n              <Name>Name</Name>\n              <Val>ValvePV1</Val>\n</String>\n            <Array>\n              <Name>Route</Name>\n              <Dimsize>2</Dimsize>\n              <String>\n                <Name>String</Name>\n                <Val>M2L:3:15:1</Val>\n</String>\n              <String>\n                <Name>String</Name>\n                <Val>M2H:1:8:1</Val>\n</String>\n</Array>\n            <Array>\n              <Name>UnRoute</Name>\n              <Dimsize>2</Dimsize>\n              <String>\n                <Name>String</Name>\n                <Val>M2L:3:15:0</Val>\n</String>\n              <String>\n                <Name>String</Name>\n                <Val>M2H:1:8:0</Val>\n</String>\n</Array>\n            <String>\n              <Name>Description</Name>\n              <Val>ValvePV1 to DMM</Val>\n</String>\n            <String>\n              <Name>Group</Name>\n              <Val>Voltages</Val>\n</String>\n            <Boolean>\n              <Name>IsGroup</Name>\n              <Val>0</Val>\n</Boolean>\n</Cluster>\n          <Cluster>\n            <Name>Alias</Name>\n            <NumElts>6</NumElts>\n            <String>\n              <Name>Name</Name>\n              <Val>ValvePV2</Val>\n</String>\n            <Array>\n              <Name>Route</Name>\n              <Dimsize>2</Dimsize>\n              <String>\n                <Name>String</Name>\n                <Val>M2H:3:16:1</Val>\n</String>\n              <String>\n                <Name>String</Name>\n                <Val>M2H:1:8:1</Val>\n</String>\n</Array>\n            <Array>\n              <Name>UnRoute</Name>\n              <Dimsize>2</Dimsize>\n              <String>\n                <Name>String</Name>\n                <Val>M2H:3:16:0</Val>\n</String>\n              <String>\n                <Name>String</Name>\n                <Val>M2H:1:8:0</Val>\n</String>\n</Array>\n            <String>\n              <Name>Description</Name>\n              <Val>ValvePV2 to DMM</Val>\n</String>\n            <String>\n              <Name>Group</Name>\n              <Val>Voltages</Val>\n</String>\n            <Boolean>\n              <Name>IsGroup</Name>\n              <Val>0</Val>\n</Boolean>\n</Cluster>\n          <Cluster>\n            <Name>Alias</Name>\n            <NumElts>6</NumElts>\n            <String>\n              <Name>Name</Name>\n              <Val>Fan</Val>\n</String>\n            <Array>\n              <Name>Route</Name>\n              <Dimsize>2</Dimsize>\n              <String>\n                <Name>String</Name>\n                <Val>M2L:3:16:1</Val>\n</String>\n              <String>\n                <Name>String</Name>\n                <Val>M2H:1:8:1</Val>\n</String>\n</Array>\n            <Array>\n              <Name>UnRoute</Name>\n              <Dimsize>2</Dimsize>\n              <String>\n                <Name>String</Name>\n                <Val>M2L:3:16:0</Val>\n</String>\n              <String>\n                <Name>String</Name>\n                <Val>M2H:1:8:0</Val>\n</String>\n</Array>\n            <String>\n              <Name>Description</Name>\n              <Val>Fan to DMM</Val>\n</String>\n            <String>\n              <Name>Group</Name>\n              <Val>Voltages</Val>\n</String>\n            <Boolean>\n              <Name>IsGroup</Name>\n              <Val>0</Val>\n</Boolean>\n</Cluster>\n          <Cluster>\n            <Name>Alias</Name>\n            <NumElts>6</NumElts>\n            <String>\n              <Name>Name</Name>\n              <Val>LCD_VCC</Val>\n</String>\n            <Array>\n              <Name>Route</Name>\n              <Dimsize>2</Dimsize>\n              <String>\n                <Name>String</Name>\n                <Val>M2L:1:18:1</Val>\n</String>\n              <String>\n                <Name>String</Name>\n                <Val>M2H:1:8:1</Val>\n</String>\n</Array>\n            <Array>\n              <Name>UnRoute</Name>\n              <Dimsize>2</Dimsize>\n              <String>\n                <Name>String</Name>\n                <Val>M2L:1:18:0</Val>\n</String>\n              <String>\n                <Name>String</Name>\n                <Val>M2H:1:8:0</Val>\n</String>\n</Array>\n            <String>\n              <Name>Description</Name>\n              <Val>LCD VCC to DMM</Val>\n</String>\n            <String>\n              <Name>Group</Name>\n              <Val>Voltages</Val>\n</String>\n            <Boolean>\n              <Name>IsGroup</Name>\n              <Val>0</Val>\n</Boolean>\n</Cluster>\n          <Cluster>\n            <Name>Alias</Name>\n            <NumElts>6</NumElts>\n            <String>\n              <Name>Name</Name>\n              <Val>ADCIN</Val>\n</String>\n            <Array>\n              <Name>Route</Name>\n              <Dimsize>2</Dimsize>\n              <String>\n                <Name>String</Name>\n                <Val>M2H:1:19:1</Val>\n</String>\n              <String>\n                <Name>String</Name>\n                <Val>M2H:1:8:1</Val>\n</String>\n</Array>\n            <Array>\n              <Name>UnRoute</Name>\n              <Dimsize>2</Dimsize>\n              <String>\n                <Name>String</Name>\n                <Val>M2H:1:19:0</Val>\n</String>\n              <String>\n                <Name>String</Name>\n                <Val>M2H:1:8:0</Val>\n</String>\n</Array>\n            <String>\n              <Name>Description</Name>\n              <Val>ADCIN to DMM</Val>\n</String>\n            <String>\n              <Name>Group</Name>\n              <Val>Voltages</Val>\n</String>\n            <Boolean>\n              <Name>IsGroup</Name>\n              <Val>0</Val>\n</Boolean>\n</Cluster>\n          <Cluster>\n            <Name>Alias</Name>\n            <NumElts>6</NumElts>\n            <String>\n              <Name>Name</Name>\n              <Val>Button_LED_1</Val>\n</String>\n            <Array>\n              <Name>Route</Name>\n              <Dimsize>2</Dimsize>\n              <String>\n                <Name>String</Name>\n                <Val>M2H:1:4:1</Val>\n</String>\n              <String>\n                <Name>String</Name>\n                <Val>M2H:3:17:1</Val>\n</String>\n</Array>\n            <Array>\n              <Name>UnRoute</Name>\n              <Dimsize>2</Dimsize>\n              <String>\n                <Name>String</Name>\n                <Val>M2H:1:4:0</Val>\n</String>\n              <String>\n                <Name>String</Name>\n                <Val>M2H:3:17:0</Val>\n</String>\n</Array>\n            <String>\n              <Name>Description</Name>\n              <Val>Button_LED_1 to DMM</Val>\n</String>\n            <String>\n              <Name>Group</Name>\n              <Val>Voltages</Val>\n</String>\n            <Boolean>\n              <Name>IsGroup</Name>\n              <Val>0</Val>\n</Boolean>\n</Cluster>\n          <Cluster>\n            <Name>Alias</Name>\n            <NumElts>6</NumElts>\n            <String>\n              <Name>Name</Name>\n              <Val>Button_LED_2</Val>\n</String>\n            <Array>\n              <Name>Route</Name>\n              <Dimsize>2</Dimsize>\n              <String>\n                <Name>String</Name>\n                <Val>M2H:1:4:1</Val>\n</String>\n              <String>\n                <Name>String</Name>\n                <Val>M2L:3:17:1</Val>\n</String>\n</Array>\n            <Array>\n              <Name>UnRoute</Name>\n              <Dimsize>2</Dimsize>\n              <String>\n                <Name>String</Name>\n                <Val>M2H:1:4:0</Val>\n</String>\n              <String>\n                <Name>String</Name>\n                <Val>M2L:3:17:0</Val>\n</String>\n</Array>\n            <String>\n              <Name>Description</Name>\n              <Val>Button_LED_2 to DMM</Val>\n</String>\n            <String>\n              <Name>Group</Name>\n              <Val>Voltages</Val>\n</String>\n            <Boolean>\n              <Name>IsGroup</Name>\n              <Val>0</Val>\n</Boolean>\n</Cluster>\n          <Cluster>\n            <Name>Alias</Name>\n            <NumElts>6</NumElts>\n            <String>\n              <Name>Name</Name>\n              <Val>Button_LED_3</Val>\n</String>\n            <Array>\n              <Name>Route</Name>\n              <Dimsize>2</Dimsize>\n              <String>\n                <Name>String</Name>\n                <Val>M2H:1:4:1</Val>\n</String>\n              <String>\n                <Name>String</Name>\n                <Val>M2H:3:18:1</Val>\n</String>\n</Array>\n            <Array>\n              <Name>UnRoute</Name>\n              <Dimsize>2</Dimsize>\n              <String>\n                <Name>String</Name>\n                <Val>M2H:1:4:0</Val>\n</String>\n              <String>\n                <Name>String</Name>\n                <Val>M2H:3:18:0</Val>\n</String>\n</Array>\n            <String>\n              <Name>Description</Name>\n              <Val>Button_LED_3 to DMM</Val>\n</String>\n            <String>\n              <Name>Group</Name>\n              <Val>Voltages</Val>\n</String>\n            <Boolean>\n              <Name>IsGroup</Name>\n              <Val>0</Val>\n</Boolean>\n</Cluster>\n</Array>\n        <Boolean>\n          <Name>Sim</Name>\n          <Val>1</Val>\n</Boolean>\n</Config>      <Ancestors>\n        <Ancestor>\n          <Class>SwitchBase</Class>\n          <Config>\n            <NumElts>1</NumElts>\n            <String>\n              <Name>default</Name>\n              <Val/>\n</String>\n</Config>        </Ancestor>\n      </Ancestors>\n    </Object>\n    <Object>\n      <Name>Matrix_2</Name>\n      <Class>Switch_Keysight_34934A</Class>\n      <Config>\n        <NumElts>4</NumElts>\n        <Refnum>\n          <Name>VISA</Name>\n          <RefKind>VISA</RefKind>\n          <Val>USB0::0x0957::0x0507::MY56485422::INSTR</Val>\n</Refnum>\n        <I32>\n          <Name>Slot</Name>\n          <Val>5</Val>\n</I32>\n        <Array>\n          <Name>SwitchMap</Name>\n          <Dimsize>59</Dimsize>\n          <Cluster>\n            <Name>Alias</Name>\n            <NumElts>6</NumElts>\n            <String>\n              <Name>Name</Name>\n              <Val>Active_Tests</Val>\n</String>\n            <Array>\n              <Name>Route</Name>\n              <Dimsize>0</Dimsize>\n              <String>\n                <Name>String</Name>\n                <Val/>\n</String>\n</Array>\n            <Array>\n              <Name>UnRoute</Name>\n              <Dimsize>0</Dimsize>\n              <String>\n                <Name>String</Name>\n                <Val/>\n</String>\n</Array>\n            <String>\n              <Name>Description</Name>\n              <Val>Tests under power</Val>\n</String>\n            <String>\n              <Name>Group</Name>\n              <Val/>\n</String>\n            <Boolean>\n              <Name>IsGroup</Name>\n              <Val>1</Val>\n</Boolean>\n</Cluster>\n          <Cluster>\n            <Name>Alias</Name>\n            <NumElts>6</NumElts>\n            <String>\n              <Name>Name</Name>\n              <Val>Power</Val>\n</String>\n            <Array>\n              <Name>Route</Name>\n              <Dimsize>0</Dimsize>\n              <String>\n                <Name>String</Name>\n                <Val/>\n</String>\n</Array>\n            <Array>\n              <Name>UnRoute</Name>\n              <Dimsize>0</Dimsize>\n              <String>\n                <Name>String</Name>\n                <Val/>\n</String>\n</Array>\n            <String>\n              <Name>Description</Name>\n              <Val>Power and Switch Control</Val>\n</String>\n            <String>\n              <Name>Group</Name>\n              <Val>Active_Tests</Val>\n</String>\n            <Boolean>\n              <Name>IsGroup</Name>\n              <Val>1</Val>\n</Boolean>\n</Cluster>\n          <Cluster>\n            <Name>Alias</Name>\n            <NumElts>6</NumElts>\n            <String>\n              <Name>Name</Name>\n              <Val>24V_Input_Relay</Val>\n</String>\n            <Array>\n              <Name>Route</Name>\n              <Dimsize>7</Dimsize>\n              <String>\n                <Name>String</Name>\n                <Val>M2L:2:1:0</Val>\n</String>\n              <String>\n                <Name>String</Name>\n                <Val>M2L:2:2:0</Val>\n</String>\n              <String>\n                <Name>String</Name>\n                <Val>M2H:2:1:1</Val>\n</String>\n              <String>\n                <Name>String</Name>\n                <Val>M2H:2:2:1</Val>\n</String>\n              <String>\n                <Name>String</Name>\n                <Val>wait:300</Val>\n</String>\n              <String>\n                <Name>String</Name>\n                <Val>M2H:2:2:0</Val>\n</String>\n              <String>\n                <Name>String</Name>\n                <Val>M2H:2:1:0</Val>\n</String>\n</Array>\n            <Array>\n              <Name>UnRoute</Name>\n              <Dimsize>7</Dimsize>\n              <String>\n                <Name>String</Name>\n                <Val>M2H:2:1:0</Val>\n</String>\n              <String>\n                <Name>String</Name>\n                <Val>M2H:2:2:0</Val>\n</String>\n              <String>\n                <Name>String</Name>\n                <Val>M2L:2:1:1</Val>\n</String>\n              <String>\n                <Name>String</Name>\n                <Val>M2L:2:2:1</Val>\n</String>\n              <String>\n                <Name>String</Name>\n                <Val>wait:300</Val>\n</String>\n              <String>\n                <Name>String</Name>\n                <Val>M2L:2:2:0</Val>\n</String>\n              <String>\n                <Name>String</Name>\n                <Val>M2L:2:1:0</Val>\n</String>\n</Array>\n            <String>\n              <Name>Description</Name>\n              <Val>Controls relay for 24V input</Val>\n</String>\n            <String>\n              <Name>Group</Name>\n              <Val>Power</Val>\n</String>\n            <Boolean>\n              <Name>IsGroup</Name>\n              <Val>0</Val>\n</Boolean>\n</Cluster>\n          <Cluster>\n            <Name>Alias</Name>\n            <NumElts>6</NumElts>\n            <String>\n              <Name>Name</Name>\n              <Val>PowerSwitch_Relay</Val>\n</String>\n            <Array>\n              <Name>Route</Name>\n              <Dimsize>7</Dimsize>\n              <String>\n                <Name>String</Name>\n                <Val>M2L:2:1:0</Val>\n</String>\n              <String>\n                <Name>String</Name>\n                <Val>M2L:2:3:0</Val>\n</String>\n              <String>\n                <Name>String</Name>\n                <Val>M2H:2:1:1</Val>\n</String>\n              <String>\n                <Name>String</Name>\n                <Val>M2H:2:3:1</Val>\n</String>\n              <String>\n                <Name>String</Name>\n                <Val>wait:300</Val>\n</String>\n              <String>\n                <Name>String</Name>\n                <Val>M2H:2:3:0</Val>\n</String>\n              <String>\n                <Name>String</Name>\n                <Val>M2H:2:1:0</Val>\n</String>\n</Array>\n            <Array>\n              <Name>UnRoute</Name>\n              <Dimsize>7</Dimsize>\n              <String>\n                <Name>String</Name>\n                <Val>M2H:2:1:0</Val>\n</String>\n              <String>\n                <Name>String</Name>\n                <Val>M2H:2:3:0</Val>\n</String>\n              <String>\n                <Name>String</Name>\n                <Val>M2L:2:1:1</Val>\n</String>\n              <String>\n                <Name>String</Name>\n                <Val>M2L:2:3:1</Val>\n</String>\n              <String>\n                <Name>String</Name>\n                <Val>wait:300</Val>\n</String>\n              <String>\n                <Name>String</Name>\n                <Val>M2L:2:3:0</Val>\n</String>\n              <String>\n                <Name>String</Name>\n                <Val>M2L:2:1:0</Val>\n</String>\n</Array>\n            <String>\n              <Name>Description</Name>\n              <Val>Controls relay for Power Switch</Val>\n</String>\n            <String>\n              <Name>Group</Name>\n              <Val>Power</Val>\n</String>\n            <Boolean>\n              <Name>IsGroup</Name>\n              <Val>0</Val>\n</Boolean>\n</Cluster>\n          <Cluster>\n            <Name>Alias</Name>\n            <NumElts>6</NumElts>\n            <String>\n              <Name>Name</Name>\n              <Val>Voltages</Val>\n</String>\n            <Array>\n              <Name>Route</Name>\n              <Dimsize>0</Dimsize>\n              <String>\n                <Name>String</Name>\n                <Val/>\n</String>\n</Array>\n            <Array>\n              <Name>UnRoute</Name>\n              <Dimsize>0</Dimsize>\n              <String>\n                <Name>String</Name>\n                <Val/>\n</String>\n</Array>\n            <String>\n              <Name>Description</Name>\n              <Val>Connect test points to DMM</Val>\n</String>\n            <String>\n              <Name>Group</Name>\n              <Val>Active_Tests</Val>\n</String>\n            <Boolean>\n              <Name>IsGroup</Name>\n              <Val>1</Val>\n</Boolean>\n</Cluster>\n          <Cluster>\n            <Name>Alias</Name>\n            <NumElts>6</NumElts>\n            <String>\n              <Name>Name</Name>\n              <Val>AUDIO_nEN</Val>\n</String>\n            <Array>\n              <Name>Route</Name>\n              <Dimsize>2</Dimsize>\n              <String>\n                <Name>String</Name>\n                <Val>M2H:1:5:1</Val>\n</String>\n              <String>\n                <Name>String</Name>\n                <Val>M2H:3:1:1</Val>\n</String>\n</Array>\n            <Array>\n              <Name>UnRoute</Name>\n              <Dimsize>2</Dimsize>\n              <String>\n                <Name>String</Name>\n                <Val>M2H:1:5:0</Val>\n</String>\n              <String>\n                <Name>String</Name>\n                <Val>M2H:3:1:0</Val>\n</String>\n</Array>\n            <String>\n              <Name>Description</Name>\n              <Val>Audio_nEN to DMM</Val>\n</String>\n            <String>\n              <Name>Group</Name>\n              <Val>Voltages</Val>\n</String>\n            <Boolean>\n              <Name>IsGroup</Name>\n              <Val>0</Val>\n</Boolean>\n</Cluster>\n          <Cluster>\n            <Name>Alias</Name>\n            <NumElts>6</NumElts>\n            <String>\n              <Name>Name</Name>\n              <Val>Audio</Val>\n</String>\n            <Array>\n              <Name>Route</Name>\n              <Dimsize>2</Dimsize>\n              <String>\n                <Name>String</Name>\n                <Val>M2H:1:6:1</Val>\n</String>\n              <String>\n                <Name>String</Name>\n                <Val>M2L:3:6:1</Val>\n</String>\n</Array>\n            <Array>\n              <Name>UnRoute</Name>\n              <Dimsize>2</Dimsize>\n              <String>\n                <Name>String</Name>\n                <Val>M2H:1:6:0</Val>\n</String>\n              <String>\n                <Name>String</Name>\n                <Val>M2L:3:6:0</Val>\n</String>\n</Array>\n            <String>\n              <Name>Description</Name>\n              <Val>Audio to DMM</Val>\n</String>\n            <String>\n              <Name>Group</Name>\n              <Val>Voltages</Val>\n</String>\n            <Boolean>\n              <Name>IsGroup</Name>\n              <Val>0</Val>\n</Boolean>\n</Cluster>\n          <Cluster>\n            <Name>Alias</Name>\n            <NumElts>6</NumElts>\n            <String>\n              <Name>Name</Name>\n              <Val>Sensors</Val>\n</String>\n            <Array>\n              <Name>Route</Name>\n              <Dimsize>0</Dimsize>\n              <String>\n                <Name>String</Name>\n                <Val/>\n</String>\n</Array>\n            <Array>\n              <Name>UnRoute</Name>\n              <Dimsize>0</Dimsize>\n              <String>\n                <Name>String</Name>\n                <Val/>\n</String>\n</Array>\n            <String>\n              <Name>Description</Name>\n              <Val>Sensor Switching</Val>\n</String>\n            <String>\n              <Name>Group</Name>\n              <Val>Active_Tests</Val>\n</String>\n            <Boolean>\n              <Name>IsGroup</Name>\n              <Val>1</Val>\n</Boolean>\n</Cluster>\n          <Cluster>\n            <Name>Alias</Name>\n            <NumElts>6</NumElts>\n            <String>\n              <Name>Name</Name>\n              <Val>Sensor_Power</Val>\n</String>\n            <Array>\n              <Name>Route</Name>\n              <Dimsize>4</Dimsize>\n              <String>\n                <Name>String</Name>\n                <Val>M1H:2:27:1</Val>\n</String>\n              <String>\n                <Name>String</Name>\n                <Val>M1H:4:1:1</Val>\n</String>\n              <String>\n                <Name>String</Name>\n                <Val>M1H:4:28:1</Val>\n</String>\n              <String>\n                <Name>String</Name>\n                <Val>M1L:2:27:1</Val>\n</String>\n</Array>\n            <Array>\n              <Name>UnRoute</Name>\n              <Dimsize>4</Dimsize>\n              <String>\n                <Name>String</Name>\n                <Val>M1H:2:27:0</Val>\n</String>\n              <String>\n                <Name>String</Name>\n                <Val>M1H:4:1:0</Val>\n</String>\n              <String>\n                <Name>String</Name>\n                <Val>M1H:4:28:0</Val>\n</String>\n              <String>\n                <Name>String</Name>\n                <Val>M1L:2:27:0</Val>\n</String>\n</Array>\n            <String>\n              <Name>Description</Name>\n              <Val>Connects sensor to power supply</Val>\n</String>\n            <String>\n              <Name>Group</Name>\n              <Val>Sensors</Val>\n</String>\n            <Boolean>\n              <Name>IsGroup</Name>\n              <Val>0</Val>\n</Boolean>\n</Cluster>\n          <Cluster>\n            <Name>Alias</Name>\n            <NumElts>6</NumElts>\n            <String>\n              <Name>Name</Name>\n              <Val>Pressure_1</Val>\n</String>\n            <Array>\n              <Name>Route</Name>\n              <Dimsize>1</Dimsize>\n              <String>\n                <Name>String</Name>\n                <Val>M1H:2:2:1</Val>\n</String>\n</Array>\n            <Array>\n              <Name>UnRoute</Name>\n              <Dimsize>1</Dimsize>\n              <String>\n                <Name>String</Name>\n                <Val>M1H:2:2:0</Val>\n</String>\n</Array>\n            <String>\n              <Name>Description</Name>\n              <Val>Pressure Sensor 1</Val>\n</String>\n            <String>\n              <Name>Group</Name>\n              <Val>Sensors</Val>\n</String>\n            <Boolean>\n              <Name>IsGroup</Name>\n              <Val>0</Val>\n</Boolean>\n</Cluster>\n          <Cluster>\n            <Name>Alias</Name>\n            <NumElts>6</NumElts>\n            <String>\n              <Name>Name</Name>\n              <Val>Pressure_2</Val>\n</String>\n            <Array>\n              <Name>Route</Name>\n              <Dimsize>1</Dimsize>\n              <String>\n                <Name>String</Name>\n                <Val>M1L:2:2:1</Val>\n</String>\n</Array>\n            <Array>\n              <Name>UnRoute</Name>\n              <Dimsize>1</Dimsize>\n              <String>\n                <Name>String</Name>\n                <Val>M1L:2:2:0</Val>\n</String>\n</Array>\n            <String>\n              <Name>Description</Name>\n              <Val>Pressure Sensor 2</Val>\n</String>\n            <String>\n              <Name>Group</Name>\n              <Val>Sensors</Val>\n</String>\n            <Boolean>\n              <Name>IsGroup</Name>\n              <Val>0</Val>\n</Boolean>\n</Cluster>\n          <Cluster>\n            <Name>Alias</Name>\n            <NumElts>6</NumElts>\n            <String>\n              <Name>Name</Name>\n              <Val>Pressure_3</Val>\n</String>\n            <Array>\n              <Name>Route</Name>\n              <Dimsize>1</Dimsize>\n              <String>\n                <Name>String</Name>\n                <Val>M1H:2:3:1</Val>\n</String>\n</Array>\n            <Array>\n              <Name>UnRoute</Name>\n              <Dimsize>1</Dimsize>\n              <String>\n                <Name>String</Name>\n                <Val>M1H:2:3:0</Val>\n</String>\n</Array>\n            <String>\n              <Name>Description</Name>\n              <Val>Pressure Sensor 3</Val>\n</String>\n            <String>\n              <Name>Group</Name>\n              <Val>Sensors</Val>\n</String>\n            <Boolean>\n              <Name>IsGroup</Name>\n              <Val>0</Val>\n</Boolean>\n</Cluster>\n          <Cluster>\n            <Name>Alias</Name>\n            <NumElts>6</NumElts>\n            <String>\n              <Name>Name</Name>\n              <Val>Pressure_4</Val>\n</String>\n            <Array>\n              <Name>Route</Name>\n              <Dimsize>1</Dimsize>\n              <String>\n                <Name>String</Name>\n                <Val>M1H:2:3:1</Val>\n</String>\n</Array>\n            <Array>\n              <Name>UnRoute</Name>\n              <Dimsize>1</Dimsize>\n              <String>\n                <Name>String</Name>\n                <Val>M1H:2:3:0</Val>\n</String>\n</Array>\n            <String>\n              <Name>Description</Name>\n              <Val>Pressure Sensor 4</Val>\n</String>\n            <String>\n              <Name>Group</Name>\n              <Val>Sensors</Val>\n</String>\n            <Boolean>\n              <Name>IsGroup</Name>\n              <Val>0</Val>\n</Boolean>\n</Cluster>\n          <Cluster>\n            <Name>Alias</Name>\n            <NumElts>6</NumElts>\n            <String>\n              <Name>Name</Name>\n              <Val>Pressure_5</Val>\n</String>\n            <Array>\n              <Name>Route</Name>\n              <Dimsize>1</Dimsize>\n              <String>\n                <Name>String</Name>\n                <Val>M1H:2:4:1</Val>\n</String>\n</Array>\n            <Array>\n              <Name>UnRoute</Name>\n              <Dimsize>1</Dimsize>\n              <String>\n                <Name>String</Name>\n                <Val>M1H:2:4:0</Val>\n</String>\n</Array>\n            <String>\n              <Name>Description</Name>\n              <Val>Pressure Sensor 5</Val>\n</String>\n            <String>\n              <Name>Group</Name>\n              <Val>Sensors</Val>\n</String>\n            <Boolean>\n              <Name>IsGroup</Name>\n              <Val>0</Val>\n</Boolean>\n</Cluster>\n          <Cluster>\n            <Name>Alias</Name>\n            <NumElts>6</NumElts>\n            <String>\n              <Name>Name</Name>\n              <Val>Pressure_6</Val>\n</String>\n            <Array>\n              <Name>Route</Name>\n              <Dimsize>1</Dimsize>\n              <String>\n                <Name>String</Name>\n                <Val>M1L:2:4:1</Val>\n</String>\n</Array>\n            <Array>\n              <Name>UnRoute</Name>\n              <Dimsize>1</Dimsize>\n              <String>\n                <Name>String</Name>\n                <Val>M1L:2:4:0</Val>\n</String>\n</Array>\n            <String>\n              <Name>Description</Name>\n              <Val>Pressure Sensor 6</Val>\n</String>\n            <String>\n              <Name>Group</Name>\n              <Val>Sensors</Val>\n</String>\n            <Boolean>\n              <Name>IsGroup</Name>\n              <Val>0</Val>\n</Boolean>\n</Cluster>\n          <Cluster>\n            <Name>Alias</Name>\n            <NumElts>6</NumElts>\n            <String>\n              <Name>Name</Name>\n              <Val>Pressure_7</Val>\n</String>\n            <Array>\n              <Name>Route</Name>\n              <Dimsize>1</Dimsize>\n              <String>\n                <Name>String</Name>\n                <Val>M1H:2:5:1</Val>\n</String>\n</Array>\n            <Array>\n              <Name>UnRoute</Name>\n              <Dimsize>1</Dimsize>\n              <String>\n                <Name>String</Name>\n                <Val>M1H:2:5:0</Val>\n</String>\n</Array>\n            <String>\n              <Name>Description</Name>\n              <Val>Pressure Sensor 7</Val>\n</String>\n            <String>\n              <Name>Group</Name>\n              <Val>Sensors</Val>\n</String>\n            <Boolean>\n              <Name>IsGroup</Name>\n              <Val>0</Val>\n</Boolean>\n</Cluster>\n          <Cluster>\n            <Name>Alias</Name>\n            <NumElts>6</NumElts>\n            <String>\n              <Name>Name</Name>\n              <Val>Pressure_8</Val>\n</String>\n            <Array>\n              <Name>Route</Name>\n              <Dimsize>1</Dimsize>\n              <String>\n                <Name>String</Name>\n                <Val>M1L:2:5:1</Val>\n</String>\n</Array>\n            <Array>\n              <Name>UnRoute</Name>\n              <Dimsize>1</Dimsize>\n              <String>\n                <Name>String</Name>\n                <Val>M1L:2:5:0</Val>\n</String>\n</Array>\n            <String>\n              <Name>Description</Name>\n              <Val>Pressure Sensor 8</Val>\n</String>\n            <String>\n              <Name>Group</Name>\n              <Val>Sensors</Val>\n</String>\n            <Boolean>\n              <Name>IsGroup</Name>\n              <Val>0</Val>\n</Boolean>\n</Cluster>\n          <Cluster>\n            <Name>Alias</Name>\n            <NumElts>6</NumElts>\n            <String>\n              <Name>Name</Name>\n              <Val>Pressure_Large</Val>\n</String>\n            <Array>\n              <Name>Route</Name>\n              <Dimsize>1</Dimsize>\n              <String>\n                <Name>String</Name>\n                <Val>M1H:2:6:1</Val>\n</String>\n</Array>\n            <Array>\n              <Name>UnRoute</Name>\n              <Dimsize>1</Dimsize>\n              <String>\n                <Name>String</Name>\n                <Val>M1H:2:6:0</Val>\n</String>\n</Array>\n            <String>\n              <Name>Description</Name>\n              <Val>Pressure Sensor Large</Val>\n</String>\n            <String>\n              <Name>Group</Name>\n              <Val>Sensors</Val>\n</String>\n            <Boolean>\n              <Name>IsGroup</Name>\n              <Val>0</Val>\n</Boolean>\n</Cluster>\n          <Cluster>\n            <Name>Alias</Name>\n            <NumElts>6</NumElts>\n            <String>\n              <Name>Name</Name>\n              <Val>Pressure_Drain</Val>\n</String>\n            <Array>\n              <Name>Route</Name>\n              <Dimsize>1</Dimsize>\n              <String>\n                <Name>String</Name>\n                <Val>M1L:2:6:1</Val>\n</String>\n</Array>\n            <Array>\n              <Name>UnRoute</Name>\n              <Dimsize>1</Dimsize>\n              <String>\n                <Name>String</Name>\n                <Val>M1L:2:6:0</Val>\n</String>\n</Array>\n            <String>\n              <Name>Description</Name>\n              <Val>Pressure Sensor Drain</Val>\n</String>\n            <String>\n              <Name>Group</Name>\n              <Val>Sensors</Val>\n</String>\n            <Boolean>\n              <Name>IsGroup</Name>\n              <Val>0</Val>\n</Boolean>\n</Cluster>\n          <Cluster>\n            <Name>Alias</Name>\n            <NumElts>6</NumElts>\n            <String>\n              <Name>Name</Name>\n              <Val>Pressure_Boost</Val>\n</String>\n            <Array>\n              <Name>Route</Name>\n              <Dimsize>1</Dimsize>\n              <String>\n                <Name>String</Name>\n                <Val>M1H:2:7:1</Val>\n</String>\n</Array>\n            <Array>\n              <Name>UnRoute</Name>\n              <Dimsize>1</Dimsize>\n              <String>\n                <Name>String</Name>\n                <Val>M1H:2:7:0</Val>\n</String>\n</Array>\n            <String>\n              <Name>Description</Name>\n              <Val>Pressure Sensor Boost</Val>\n</String>\n            <String>\n              <Name>Group</Name>\n              <Val>Sensors</Val>\n</String>\n            <Boolean>\n              <Name>IsGroup</Name>\n              <Val>0</Val>\n</Boolean>\n</Cluster>\n          <Cluster>\n            <Name>Alias</Name>\n            <NumElts>6</NumElts>\n            <String>\n              <Name>Name</Name>\n              <Val>Pressure_FS</Val>\n</String>\n            <Array>\n              <Name>Route</Name>\n              <Dimsize>1</Dimsize>\n              <String>\n                <Name>String</Name>\n                <Val>M1L:2:7:1</Val>\n</String>\n</Array>\n            <Array>\n              <Name>UnRoute</Name>\n              <Dimsize>1</Dimsize>\n              <String>\n                <Name>String</Name>\n                <Val>M1L:2:7:0</Val>\n</String>\n</Array>\n            <String>\n              <Name>Description</Name>\n              <Val>Pressure Sensor FS</Val>\n</String>\n            <String>\n              <Name>Group</Name>\n              <Val>Sensors</Val>\n</String>\n            <Boolean>\n              <Name>IsGroup</Name>\n              <Val>0</Val>\n</Boolean>\n</Cluster>\n          <Cluster>\n            <Name>Alias</Name>\n            <NumElts>6</NumElts>\n            <String>\n              <Name>Name</Name>\n              <Val>Pressure_FL</Val>\n</String>\n            <Array>\n              <Name>Route</Name>\n              <Dimsize>1</Dimsize>\n              <String>\n                <Name>String</Name>\n                <Val>M1H:2:8:1</Val>\n</String>\n</Array>\n            <Array>\n              <Name>UnRoute</Name>\n              <Dimsize>1</Dimsize>\n              <String>\n                <Name>String</Name>\n                <Val>M1H:2:8:0</Val>\n</String>\n</Array>\n            <String>\n              <Name>Description</Name>\n              <Val>Pressure Sensor FL</Val>\n</String>\n            <String>\n              <Name>Group</Name>\n              <Val>Sensors</Val>\n</String>\n            <Boolean>\n              <Name>IsGroup</Name>\n              <Val>0</Val>\n</Boolean>\n</Cluster>\n          <Cluster>\n            <Name>Alias</Name>\n            <NumElts>6</NumElts>\n            <String>\n              <Name>Name</Name>\n              <Val>Pressure_Small</Val>\n</String>\n            <Array>\n              <Name>Route</Name>\n              <Dimsize>1</Dimsize>\n              <String>\n                <Name>String</Name>\n                <Val>M1L:2:8:1</Val>\n</String>\n</Array>\n            <Array>\n              <Name>UnRoute</Name>\n              <Dimsize>1</Dimsize>\n              <String>\n                <Name>String</Name>\n                <Val>M1L:2:8:0</Val>\n</String>\n</Array>\n            <String>\n              <Name>Description</Name>\n              <Val>Pressure Sensor Small</Val>\n</String>\n            <String>\n              <Name>Group</Name>\n              <Val>Sensors</Val>\n</String>\n            <Boolean>\n              <Name>IsGroup</Name>\n              <Val>0</Val>\n</Boolean>\n</Cluster>\n          <Cluster>\n            <Name>Alias</Name>\n            <NumElts>6</NumElts>\n            <String>\n              <Name>Name</Name>\n              <Val>Temp_1</Val>\n</String>\n            <Array>\n              <Name>Route</Name>\n              <Dimsize>1</Dimsize>\n              <String>\n                <Name>String</Name>\n                <Val>M1H:2:9:1</Val>\n</String>\n</Array>\n            <Array>\n              <Name>UnRoute</Name>\n              <Dimsize>1</Dimsize>\n              <String>\n                <Name>String</Name>\n                <Val>M1H:2:9:0</Val>\n</String>\n</Array>\n            <String>\n              <Name>Description</Name>\n              <Val>Temp Sensor 1</Val>\n</String>\n            <String>\n              <Name>Group</Name>\n              <Val>Sensors</Val>\n</String>\n            <Boolean>\n              <Name>IsGroup</Name>\n              <Val>0</Val>\n</Boolean>\n</Cluster>\n          <Cluster>\n            <Name>Alias</Name>\n            <NumElts>6</NumElts>\n            <String>\n              <Name>Name</Name>\n              <Val>Temp_2</Val>\n</String>\n            <Array>\n              <Name>Route</Name>\n              <Dimsize>1</Dimsize>\n              <String>\n                <Name>String</Name>\n                <Val>M1L:2:9:1</Val>\n</String>\n</Array>\n            <Array>\n              <Name>UnRoute</Name>\n              <Dimsize>1</Dimsize>\n              <String>\n                <Name>String</Name>\n                <Val>M1L:2:9:0</Val>\n</String>\n</Array>\n            <String>\n              <Name>Description</Name>\n              <Val>Temp Sensor 2</Val>\n</String>\n            <String>\n              <Name>Group</Name>\n              <Val>Sensors</Val>\n</String>\n            <Boolean>\n              <Name>IsGroup</Name>\n              <Val>0</Val>\n</Boolean>\n</Cluster>\n          <Cluster>\n            <Name>Alias</Name>\n            <NumElts>6</NumElts>\n            <String>\n              <Name>Name</Name>\n              <Val>Temp_3</Val>\n</String>\n            <Array>\n              <Name>Route</Name>\n              <Dimsize>1</Dimsize>\n              <String>\n                <Name>String</Name>\n                <Val>M1H:2:10:1</Val>\n</String>\n</Array>\n            <Array>\n              <Name>UnRoute</Name>\n              <Dimsize>1</Dimsize>\n              <String>\n                <Name>String</Name>\n                <Val>M1H:2:10:0</Val>\n</String>\n</Array>\n            <String>\n              <Name>Description</Name>\n              <Val>Temp Sensor 3</Val>\n</String>\n            <String>\n              <Name>Group</Name>\n              <Val>Sensors</Val>\n</String>\n            <Boolean>\n              <Name>IsGroup</Name>\n              <Val>0</Val>\n</Boolean>\n</Cluster>\n          <Cluster>\n            <Name>Alias</Name>\n            <NumElts>6</NumElts>\n            <String>\n              <Name>Name</Name>\n              <Val>Paste_1</Val>\n</String>\n            <Array>\n              <Name>Route</Name>\n              <Dimsize>1</Dimsize>\n              <String>\n                <Name>String</Name>\n                <Val>M1L:2:10:1</Val>\n</String>\n</Array>\n            <Array>\n              <Name>UnRoute</Name>\n              <Dimsize>1</Dimsize>\n              <String>\n                <Name>String</Name>\n                <Val>M1L:2:10:0</Val>\n</String>\n</Array>\n            <String>\n              <Name>Description</Name>\n              <Val>Paste Sensor 1</Val>\n</String>\n            <String>\n              <Name>Group</Name>\n              <Val>Sensors</Val>\n</String>\n            <Boolean>\n              <Name>IsGroup</Name>\n              <Val>0</Val>\n</Boolean>\n</Cluster>\n          <Cluster>\n            <Name>Alias</Name>\n            <NumElts>6</NumElts>\n            <String>\n              <Name>Name</Name>\n              <Val>Paste_2</Val>\n</String>\n            <Array>\n              <Name>Route</Name>\n              <Dimsize>1</Dimsize>\n              <String>\n                <Name>String</Name>\n                <Val>M1H:2:11:1</Val>\n</String>\n</Array>\n            <Array>\n              <Name>UnRoute</Name>\n              <Dimsize>1</Dimsize>\n              <String>\n                <Name>String</Name>\n                <Val>M1H:2:11:0</Val>\n</String>\n</Array>\n            <String>\n              <Name>Description</Name>\n              <Val>Paste Sensor 2</Val>\n</String>\n            <String>\n              <Name>Group</Name>\n              <Val>Sensors</Val>\n</String>\n            <Boolean>\n              <Name>IsGroup</Name>\n              <Val>0</Val>\n</Boolean>\n</Cluster>\n          <Cluster>\n            <Name>Alias</Name>\n            <NumElts>6</NumElts>\n            <String>\n              <Name>Name</Name>\n              <Val>Paste_3</Val>\n</String>\n            <Array>\n              <Name>Route</Name>\n              <Dimsize>1</Dimsize>\n              <String>\n                <Name>String</Name>\n                <Val>M1H:2:11:1</Val>\n</String>\n</Array>\n            <Array>\n              <Name>UnRoute</Name>\n              <Dimsize>1</Dimsize>\n              <String>\n                <Name>String</Name>\n                <Val>M1H:2:11:0</Val>\n</String>\n</Array>\n            <String>\n              <Name>Description</Name>\n              <Val>Paste Sensor 3</Val>\n</String>\n            <String>\n              <Name>Group</Name>\n              <Val>Sensors</Val>\n</String>\n            <Boolean>\n              <Name>IsGroup</Name>\n              <Val>0</Val>\n</Boolean>\n</Cluster>\n          <Cluster>\n            <Name>Alias</Name>\n            <NumElts>6</NumElts>\n            <String>\n              <Name>Name</Name>\n              <Val>Paste_4</Val>\n</String>\n            <Array>\n              <Name>Route</Name>\n              <Dimsize>1</Dimsize>\n              <String>\n                <Name>String</Name>\n                <Val>M1H:2:12:1</Val>\n</String>\n</Array>\n            <Array>\n              <Name>UnRoute</Name>\n              <Dimsize>1</Dimsize>\n              <String>\n                <Name>String</Name>\n                <Val>M1H:2:12:0</Val>\n</String>\n</Array>\n            <String>\n              <Name>Description</Name>\n              <Val>Paste Sensor 4</Val>\n</String>\n            <String>\n              <Name>Group</Name>\n              <Val>Sensors</Val>\n</String>\n            <Boolean>\n              <Name>IsGroup</Name>\n              <Val>0</Val>\n</Boolean>\n</Cluster>\n          <Cluster>\n            <Name>Alias</Name>\n            <NumElts>6</NumElts>\n            <String>\n              <Name>Name</Name>\n              <Val>Paste_5</Val>\n</String>\n            <Array>\n              <Name>Route</Name>\n              <Dimsize>1</Dimsize>\n              <String>\n                <Name>String</Name>\n                <Val>M1L:2:12:1</Val>\n</String>\n</Array>\n            <Array>\n              <Name>UnRoute</Name>\n              <Dimsize>1</Dimsize>\n              <String>\n                <Name>String</Name>\n                <Val>M1L:2:12:0</Val>\n</String>\n</Array>\n            <String>\n              <Name>Description</Name>\n              <Val>Paste Sensor 5</Val>\n</String>\n            <String>\n              <Name>Group</Name>\n              <Val>Sensors</Val>\n</String>\n            <Boolean>\n              <Name>IsGroup</Name>\n              <Val>0</Val>\n</Boolean>\n</Cluster>\n          <Cluster>\n            <Name>Alias</Name>\n            <NumElts>6</NumElts>\n            <String>\n              <Name>Name</Name>\n              <Val>Paste_6</Val>\n</String>\n            <Array>\n              <Name>Route</Name>\n              <Dimsize>1</Dimsize>\n              <String>\n                <Name>String</Name>\n                <Val>M1H:2:13:1</Val>\n</String>\n</Array>\n            <Array>\n              <Name>UnRoute</Name>\n              <Dimsize>1</Dimsize>\n              <String>\n                <Name>String</Name>\n                <Val>M1H:2:13:0</Val>\n</String>\n</Array>\n            <String>\n              <Name>Description</Name>\n              <Val>Paste Sensor 6</Val>\n</String>\n            <String>\n              <Name>Group</Name>\n              <Val>Sensors</Val>\n</String>\n            <Boolean>\n              <Name>IsGroup</Name>\n              <Val>0</Val>\n</Boolean>\n</Cluster>\n          <Cluster>\n            <Name>Alias</Name>\n            <NumElts>6</NumElts>\n            <String>\n              <Name>Name</Name>\n              <Val>Paste_7</Val>\n</String>\n            <Array>\n              <Name>Route</Name>\n              <Dimsize>1</Dimsize>\n              <String>\n                <Name>String</Name>\n                <Val>M1H:2:13:1</Val>\n</String>\n</Array>\n            <Array>\n              <Name>UnRoute</Name>\n              <Dimsize>1</Dimsize>\n              <String>\n                <Name>String</Name>\n                <Val>M1H:2:13:0</Val>\n</String>\n</Array>\n            <String>\n              <Name>Description</Name>\n              <Val>Paste Sensor 7</Val>\n</String>\n            <String>\n              <Name>Group</Name>\n              <Val>Sensors</Val>\n</String>\n            <Boolean>\n              <Name>IsGroup</Name>\n              <Val>0</Val>\n</Boolean>\n</Cluster>\n          <Cluster>\n            <Name>Alias</Name>\n            <NumElts>6</NumElts>\n            <String>\n              <Name>Name</Name>\n              <Val>Paste_8</Val>\n</String>\n            <Array>\n              <Name>Route</Name>\n              <Dimsize>1</Dimsize>\n              <String>\n                <Name>String</Name>\n                <Val>M1H:2:14:1</Val>\n</String>\n</Array>\n            <Array>\n              <Name>UnRoute</Name>\n              <Dimsize>1</Dimsize>\n              <String>\n                <Name>String</Name>\n                <Val>M1H:2:14:0</Val>\n</String>\n</Array>\n            <String>\n              <Name>Description</Name>\n              <Val>Paste Sensor 8</Val>\n</String>\n            <String>\n              <Name>Group</Name>\n              <Val>Sensors</Val>\n</String>\n            <Boolean>\n              <Name>IsGroup</Name>\n              <Val>0</Val>\n</Boolean>\n</Cluster>\n          <Cluster>\n            <Name>Alias</Name>\n            <NumElts>6</NumElts>\n            <String>\n              <Name>Name</Name>\n              <Val>Paste_9</Val>\n</String>\n            <Array>\n              <Name>Route</Name>\n              <Dimsize>1</Dimsize>\n              <String>\n                <Name>String</Name>\n                <Val>M1L:2:14:1</Val>\n</String>\n</Array>\n            <Array>\n              <Name>UnRoute</Name>\n              <Dimsize>1</Dimsize>\n              <String>\n                <Name>String</Name>\n                <Val>M1L:2:14:0</Val>\n</String>\n</Array>\n            <String>\n              <Name>Description</Name>\n              <Val>Paste Sensor 9</Val>\n</String>\n            <String>\n              <Name>Group</Name>\n              <Val>Sensors</Val>\n</String>\n            <Boolean>\n              <Name>IsGroup</Name>\n              <Val>0</Val>\n</Boolean>\n</Cluster>\n          <Cluster>\n            <Name>Alias</Name>\n            <NumElts>6</NumElts>\n            <String>\n              <Name>Name</Name>\n              <Val>Paste_10</Val>\n</String>\n            <Array>\n              <Name>Route</Name>\n              <Dimsize>1</Dimsize>\n              <String>\n                <Name>String</Name>\n                <Val>M1H:2:15:1</Val>\n</String>\n</Array>\n            <Array>\n              <Name>UnRoute</Name>\n              <Dimsize>1</Dimsize>\n              <String>\n                <Name>String</Name>\n                <Val>M1H:2:15:0</Val>\n</String>\n</Array>\n            <String>\n              <Name>Description</Name>\n              <Val>Paste Sensor 10</Val>\n</String>\n            <String>\n              <Name>Group</Name>\n              <Val>Sensors</Val>\n</String>\n            <Boolean>\n              <Name>IsGroup</Name>\n              <Val>0</Val>\n</Boolean>\n</Cluster>\n          <Cluster>\n            <Name>Alias</Name>\n            <NumElts>6</NumElts>\n            <String>\n              <Name>Name</Name>\n              <Val>Paste_11</Val>\n</String>\n            <Array>\n              <Name>Route</Name>\n              <Dimsize>1</Dimsize>\n              <String>\n                <Name>String</Name>\n                <Val>M1L:2:15:1</Val>\n</String>\n</Array>\n            <Array>\n              <Name>UnRoute</Name>\n              <Dimsize>1</Dimsize>\n              <String>\n                <Name>String</Name>\n                <Val>M1L:2:15:0</Val>\n</String>\n</Array>\n            <String>\n              <Name>Description</Name>\n              <Val>Paste Sensor 11</Val>\n</String>\n            <String>\n              <Name>Group</Name>\n              <Val>Sensors</Val>\n</String>\n            <Boolean>\n              <Name>IsGroup</Name>\n              <Val>0</Val>\n</Boolean>\n</Cluster>\n          <Cluster>\n            <Name>Alias</Name>\n            <NumElts>6</NumElts>\n            <String>\n              <Name>Name</Name>\n              <Val>Paste_LEDs</Val>\n</String>\n            <Array>\n              <Name>Route</Name>\n              <Dimsize>0</Dimsize>\n              <String>\n                <Name>String</Name>\n                <Val/>\n</String>\n</Array>\n            <Array>\n              <Name>UnRoute</Name>\n              <Dimsize>0</Dimsize>\n              <String>\n                <Name>String</Name>\n                <Val/>\n</String>\n</Array>\n            <String>\n              <Name>Description</Name>\n              <Val>Switches Paste LED's to DMM_I</Val>\n</String>\n            <String>\n              <Name>Group</Name>\n              <Val>Active_Tests</Val>\n</String>\n            <Boolean>\n              <Name>IsGroup</Name>\n              <Val>1</Val>\n</Boolean>\n</Cluster>\n          <Cluster>\n            <Name>Alias</Name>\n            <NumElts>6</NumElts>\n            <String>\n              <Name>Name</Name>\n              <Val>Paste_LED_DMM_I</Val>\n</String>\n            <Array>\n              <Name>Route</Name>\n              <Dimsize>2</Dimsize>\n              <String>\n                <Name>String</Name>\n                <Val>M2H:2:7:1</Val>\n</String>\n              <String>\n                <Name>String</Name>\n                <Val>M2H:2:26:1</Val>\n</String>\n</Array>\n            <Array>\n              <Name>UnRoute</Name>\n              <Dimsize>2</Dimsize>\n              <String>\n                <Name>String</Name>\n                <Val>M2H:2:7:1</Val>\n</String>\n              <String>\n                <Name>String</Name>\n                <Val>M2H:2:26:1</Val>\n</String>\n</Array>\n            <String>\n              <Name>Description</Name>\n              <Val>Connect DMM_I to switch</Val>\n</String>\n            <String>\n              <Name>Group</Name>\n              <Val>Paste_LEDs</Val>\n</String>\n            <Boolean>\n              <Name>IsGroup</Name>\n              <Val>0</Val>\n</Boolean>\n</Cluster>\n          <Cluster>\n            <Name>Alias</Name>\n            <NumElts>6</NumElts>\n            <String>\n              <Name>Name</Name>\n              <Val>Paste_LED_1</Val>\n</String>\n            <Array>\n              <Name>Route</Name>\n              <Dimsize>1</Dimsize>\n              <String>\n                <Name>String</Name>\n                <Val>M2H:3:9:1</Val>\n</String>\n</Array>\n            <Array>\n              <Name>UnRoute</Name>\n              <Dimsize>1</Dimsize>\n              <String>\n                <Name>String</Name>\n                <Val>M2H:3:9:0</Val>\n</String>\n</Array>\n            <String>\n              <Name>Description</Name>\n              <Val>Connect Paste_LED_1 to DMM_I</Val>\n</String>\n            <String>\n              <Name>Group</Name>\n              <Val>Paste_LEDs</Val>\n</String>\n            <Boolean>\n              <Name>IsGroup</Name>\n              <Val>0</Val>\n</Boolean>\n</Cluster>\n          <Cluster>\n            <Name>Alias</Name>\n            <NumElts>6</NumElts>\n            <String>\n              <Name>Name</Name>\n              <Val>Paste_LED_2</Val>\n</String>\n            <Array>\n              <Name>Route</Name>\n              <Dimsize>1</Dimsize>\n              <String>\n                <Name>String</Name>\n                <Val>M2L:3:9:1</Val>\n</String>\n</Array>\n            <Array>\n              <Name>UnRoute</Name>\n              <Dimsize>1</Dimsize>\n              <String>\n                <Name>String</Name>\n                <Val>M2L:3:9:0</Val>\n</String>\n</Array>\n            <String>\n              <Name>Description</Name>\n              <Val>Connect Paste_LED_2 to DMM_I</Val>\n</String>\n            <String>\n              <Name>Group</Name>\n              <Val>Paste_LEDs</Val>\n</String>\n            <Boolean>\n              <Name>IsGroup</Name>\n              <Val>0</Val>\n</Boolean>\n</Cluster>\n          <Cluster>\n            <Name>Alias</Name>\n            <NumElts>6</NumElts>\n            <String>\n              <Name>Name</Name>\n              <Val>Paste_LED_3</Val>\n</String>\n            <Array>\n              <Name>Route</Name>\n              <Dimsize>1</Dimsize>\n              <String>\n                <Name>String</Name>\n                <Val>M2H:3:10:1</Val>\n</String>\n</Array>\n            <Array>\n              <Name>UnRoute</Name>\n              <Dimsize>1</Dimsize>\n              <String>\n                <Name>String</Name>\n                <Val>M2H:3:10:0</Val>\n</String>\n</Array>\n            <String>\n              <Name>Description</Name>\n              <Val>Connect Paste_LED_3 to DMM_I</Val>\n</String>\n            <String>\n              <Name>Group</Name>\n              <Val>Paste_LEDs</Val>\n</String>\n            <Boolean>\n              <Name>IsGroup</Name>\n              <Val>0</Val>\n</Boolean>\n</Cluster>\n          <Cluster>\n            <Name>Alias</Name>\n            <NumElts>6</NumElts>\n            <String>\n              <Name>Name</Name>\n              <Val>Paste_LED_4</Val>\n</String>\n            <Array>\n              <Name>Route</Name>\n              <Dimsize>1</Dimsize>\n              <String>\n                <Name>String</Name>\n                <Val>M2L:3:10:1</Val>\n</String>\n</Array>\n            <Array>\n              <Name>UnRoute</Name>\n              <Dimsize>1</Dimsize>\n              <String>\n                <Name>String</Name>\n                <Val>M2L:3:10:0</Val>\n</String>\n</Array>\n            <String>\n              <Name>Description</Name>\n              <Val>Connect Paste_LED_4 to DMM_I</Val>\n</String>\n            <String>\n              <Name>Group</Name>\n              <Val>Paste_LEDs</Val>\n</String>\n            <Boolean>\n              <Name>IsGroup</Name>\n              <Val>0</Val>\n</Boolean>\n</Cluster>\n          <Cluster>\n            <Name>Alias</Name>\n            <NumElts>6</NumElts>\n            <String>\n              <Name>Name</Name>\n              <Val>Paste_LED_5</Val>\n</String>\n            <Array>\n              <Name>Route</Name>\n              <Dimsize>1</Dimsize>\n              <String>\n                <Name>String</Name>\n                <Val>M2H:3:11:1</Val>\n</String>\n</Array>\n            <Array>\n              <Name>UnRoute</Name>\n              <Dimsize>1</Dimsize>\n              <String>\n                <Name>String</Name>\n                <Val>M2H:3:11:0</Val>\n</String>\n</Array>\n            <String>\n              <Name>Description</Name>\n              <Val>Connect Paste_LED_5 to DMM_I</Val>\n</String>\n            <String>\n              <Name>Group</Name>\n              <Val>Paste_LEDs</Val>\n</String>\n            <Boolean>\n              <Name>IsGroup</Name>\n              <Val>0</Val>\n</Boolean>\n</Cluster>\n          <Cluster>\n            <Name>Alias</Name>\n            <NumElts>6</NumElts>\n            <String>\n              <Name>Name</Name>\n              <Val>Paste_LED_6</Val>\n</String>\n            <Array>\n              <Name>Route</Name>\n              <Dimsize>1</Dimsize>\n              <String>\n                <Name>String</Name>\n                <Val>M2L:3:11:1</Val>\n</String>\n</Array>\n            <Array>\n              <Name>UnRoute</Name>\n              <Dimsize>1</Dimsize>\n              <String>\n                <Name>String</Name>\n                <Val>M2L:3:11:0</Val>\n</String>\n</Array>\n            <String>\n              <Name>Description</Name>\n              <Val>Connect Paste_LED_6 to DMM_I</Val>\n</String>\n            <String>\n              <Name>Group</Name>\n              <Val>Paste_LEDs</Val>\n</String>\n            <Boolean>\n              <Name>IsGroup</Name>\n              <Val>0</Val>\n</Boolean>\n</Cluster>\n          <Cluster>\n            <Name>Alias</Name>\n            <NumElts>6</NumElts>\n            <String>\n              <Name>Name</Name>\n              <Val>Paste_LED_7</Val>\n</String>\n            <Array>\n              <Name>Route</Name>\n              <Dimsize>1</Dimsize>\n              <String>\n                <Name>String</Name>\n                <Val>M2H:3:12:1</Val>\n</String>\n</Array>\n            <Array>\n              <Name>UnRoute</Name>\n              <Dimsize>1</Dimsize>\n              <String>\n                <Name>String</Name>\n                <Val>M2H:3:12:0</Val>\n</String>\n</Array>\n            <String>\n              <Name>Description</Name>\n              <Val>Connect Paste_LED_7 to DMM_I</Val>\n</String>\n            <String>\n              <Name>Group</Name>\n              <Val>Paste_LEDs</Val>\n</String>\n            <Boolean>\n              <Name>IsGroup</Name>\n              <Val>0</Val>\n</Boolean>\n</Cluster>\n          <Cluster>\n            <Name>Alias</Name>\n            <NumElts>6</NumElts>\n            <String>\n              <Name>Name</Name>\n              <Val>Paste_LED_8</Val>\n</String>\n            <Array>\n              <Name>Route</Name>\n              <Dimsize>1</Dimsize>\n              <String>\n                <Name>String</Name>\n                <Val>M2L:3:12:1</Val>\n</String>\n</Array>\n            <Array>\n              <Name>UnRoute</Name>\n              <Dimsize>1</Dimsize>\n              <String>\n                <Name>String</Name>\n                <Val>M2L:3:12:0</Val>\n</String>\n</Array>\n            <String>\n              <Name>Description</Name>\n              <Val>Connect Paste_LED_8 to DMM_I</Val>\n</String>\n            <String>\n              <Name>Group</Name>\n              <Val>Paste_LEDs</Val>\n</String>\n            <Boolean>\n              <Name>IsGroup</Name>\n              <Val>0</Val>\n</Boolean>\n</Cluster>\n          <Cluster>\n            <Name>Alias</Name>\n            <NumElts>6</NumElts>\n            <String>\n              <Name>Name</Name>\n              <Val>Paste_LED_9</Val>\n</String>\n            <Array>\n              <Name>Route</Name>\n              <Dimsize>1</Dimsize>\n              <String>\n                <Name>String</Name>\n                <Val>M2H:3:13:1</Val>\n</String>\n</Array>\n            <Array>\n              <Name>UnRoute</Name>\n              <Dimsize>1</Dimsize>\n              <String>\n                <Name>String</Name>\n                <Val>M2H:3:13:0</Val>\n</String>\n</Array>\n            <String>\n              <Name>Description</Name>\n              <Val>Connect Paste_LED_9 to DMM_I</Val>\n</String>\n            <String>\n              <Name>Group</Name>\n              <Val>Paste_LEDs</Val>\n</String>\n            <Boolean>\n              <Name>IsGroup</Name>\n              <Val>0</Val>\n</Boolean>\n</Cluster>\n          <Cluster>\n            <Name>Alias</Name>\n            <NumElts>6</NumElts>\n            <String>\n              <Name>Name</Name>\n              <Val>Paste_LED_10</Val>\n</String>\n            <Array>\n              <Name>Route</Name>\n              <Dimsize>1</Dimsize>\n              <String>\n                <Name>String</Name>\n                <Val>M2H:3:15:1</Val>\n</String>\n</Array>\n            <Array>\n              <Name>UnRoute</Name>\n              <Dimsize>1</Dimsize>\n              <String>\n                <Name>String</Name>\n                <Val>M2H:3:15:0</Val>\n</String>\n</Array>\n            <String>\n              <Name>Description</Name>\n              <Val>Connect Paste_LED_10 to DMM_I</Val>\n</String>\n            <String>\n              <Name>Group</Name>\n              <Val>Paste_LEDs</Val>\n</String>\n            <Boolean>\n              <Name>IsGroup</Name>\n              <Val>0</Val>\n</Boolean>\n</Cluster>\n          <Cluster>\n            <Name>Alias</Name>\n            <NumElts>6</NumElts>\n            <String>\n              <Name>Name</Name>\n              <Val>Paste_LED_11</Val>\n</String>\n            <Array>\n              <Name>Route</Name>\n              <Dimsize>1</Dimsize>\n              <String>\n                <Name>String</Name>\n                <Val>M2L:3:15:1</Val>\n</String>\n</Array>\n            <Array>\n              <Name>UnRoute</Name>\n              <Dimsize>1</Dimsize>\n              <String>\n                <Name>String</Name>\n                <Val>M2L:3:15:0</Val>\n</String>\n</Array>\n            <String>\n              <Name>Description</Name>\n              <Val>Connect Paste_LED_11 to DMM_I</Val>\n</String>\n            <String>\n              <Name>Group</Name>\n              <Val>Paste_LEDs</Val>\n</String>\n            <Boolean>\n              <Name>IsGroup</Name>\n              <Val>0</Val>\n</Boolean>\n</Cluster>\n          <Cluster>\n            <Name>Alias</Name>\n            <NumElts>6</NumElts>\n            <String>\n              <Name>Name</Name>\n              <Val>Buttons</Val>\n</String>\n            <Array>\n              <Name>Route</Name>\n              <Dimsize>0</Dimsize>\n              <String>\n                <Name>String</Name>\n                <Val/>\n</String>\n</Array>\n            <Array>\n              <Name>UnRoute</Name>\n              <Dimsize>0</Dimsize>\n              <String>\n                <Name>String</Name>\n                <Val/>\n</String>\n</Array>\n            <String>\n              <Name>Description</Name>\n              <Val>Switches in the buttons</Val>\n</String>\n            <String>\n              <Name>Group</Name>\n              <Val>Active_Tests</Val>\n</String>\n            <Boolean>\n              <Name>IsGroup</Name>\n              <Val>1</Val>\n</Boolean>\n</Cluster>\n          <Cluster>\n            <Name>Alias</Name>\n            <NumElts>6</NumElts>\n            <String>\n              <Name>Name</Name>\n              <Val>Button_1</Val>\n</String>\n            <Array>\n              <Name>Route</Name>\n              <Dimsize>3</Dimsize>\n              <String>\n                <Name>String</Name>\n                <Val>M2H:2:1:1</Val>\n</String>\n              <String>\n                <Name>String</Name>\n                <Val>M2L:2:1:1</Val>\n</String>\n              <String>\n                <Name>String</Name>\n                <Val>M2L:2:14:1</Val>\n</String>\n</Array>\n            <Array>\n              <Name>UnRoute</Name>\n              <Dimsize>3</Dimsize>\n              <String>\n                <Name>String</Name>\n                <Val>M2H:2:1:0</Val>\n</String>\n              <String>\n                <Name>String</Name>\n                <Val>M2L:2:1:0</Val>\n</String>\n              <String>\n                <Name>String</Name>\n                <Val>M2L:2:14:0</Val>\n</String>\n</Array>\n            <String>\n              <Name>Description</Name>\n              <Val>Connect Button 1</Val>\n</String>\n            <String>\n              <Name>Group</Name>\n              <Val>Buttons</Val>\n</String>\n            <Boolean>\n              <Name>IsGroup</Name>\n              <Val>0</Val>\n</Boolean>\n</Cluster>\n          <Cluster>\n            <Name>Alias</Name>\n            <NumElts>6</NumElts>\n            <String>\n              <Name>Name</Name>\n              <Val>Button_2</Val>\n</String>\n            <Array>\n              <Name>Route</Name>\n              <Dimsize>3</Dimsize>\n              <String>\n                <Name>String</Name>\n                <Val>M2H:2:1:1</Val>\n</String>\n              <String>\n                <Name>String</Name>\n                <Val>M2L:2:1:1</Val>\n</String>\n              <String>\n                <Name>String</Name>\n                <Val>M2H:2:15:1</Val>\n</String>\n</Array>\n            <Array>\n              <Name>UnRoute</Name>\n              <Dimsize>3</Dimsize>\n              <String>\n                <Name>String</Name>\n                <Val>M2H:2:1:0</Val>\n</String>\n              <String>\n                <Name>String</Name>\n                <Val>M2L:2:1:0</Val>\n</String>\n              <String>\n                <Name>String</Name>\n                <Val>M2H:2:15:0</Val>\n</String>\n</Array>\n            <String>\n              <Name>Description</Name>\n              <Val>Connect Button 2</Val>\n</String>\n            <String>\n              <Name>Group</Name>\n              <Val>Buttons</Val>\n</String>\n            <Boolean>\n              <Name>IsGroup</Name>\n              <Val>0</Val>\n</Boolean>\n</Cluster>\n          <Cluster>\n            <Name>Alias</Name>\n            <NumElts>6</NumElts>\n            <String>\n              <Name>Name</Name>\n              <Val>Button_3</Val>\n</String>\n            <Array>\n              <Name>Route</Name>\n              <Dimsize>3</Dimsize>\n              <String>\n                <Name>String</Name>\n                <Val>M2H:2:1:1</Val>\n</String>\n              <String>\n                <Name>String</Name>\n                <Val>M2L:2:1:1</Val>\n</String>\n              <String>\n                <Name>String</Name>\n                <Val>M2L:2:15:1</Val>\n</String>\n</Array>\n            <Array>\n              <Name>UnRoute</Name>\n              <Dimsize>3</Dimsize>\n              <String>\n                <Name>String</Name>\n                <Val>M2H:2:1:0</Val>\n</String>\n              <String>\n                <Name>String</Name>\n                <Val>M2L:2:1:0</Val>\n</String>\n              <String>\n                <Name>String</Name>\n                <Val>M2L:2:15:0</Val>\n</String>\n</Array>\n            <String>\n              <Name>Description</Name>\n              <Val>Connect Button 3</Val>\n</String>\n            <String>\n              <Name>Group</Name>\n              <Val>Buttons</Val>\n</String>\n            <Boolean>\n              <Name>IsGroup</Name>\n              <Val>0</Val>\n</Boolean>\n</Cluster>\n          <Cluster>\n            <Name>Alias</Name>\n            <NumElts>6</NumElts>\n            <String>\n              <Name>Name</Name>\n              <Val>Button_4</Val>\n</String>\n            <Array>\n              <Name>Route</Name>\n              <Dimsize>3</Dimsize>\n              <String>\n                <Name>String</Name>\n                <Val>M2H:2:1:1</Val>\n</String>\n              <String>\n                <Name>String</Name>\n                <Val>M2L:2:1:1</Val>\n</String>\n              <String>\n                <Name>String</Name>\n                <Val>M2H:2:16:1</Val>\n</String>\n</Array>\n            <Array>\n              <Name>UnRoute</Name>\n              <Dimsize>3</Dimsize>\n              <String>\n                <Name>String</Name>\n                <Val>M2H:2:1:0</Val>\n</String>\n              <String>\n                <Name>String</Name>\n                <Val>M2L:2:1:0</Val>\n</String>\n              <String>\n                <Name>String</Name>\n                <Val>M2H:2:16:0</Val>\n</String>\n</Array>\n            <String>\n              <Name>Description</Name>\n              <Val>Connect Button 4</Val>\n</String>\n            <String>\n              <Name>Group</Name>\n              <Val>Buttons</Val>\n</String>\n            <Boolean>\n              <Name>IsGroup</Name>\n              <Val>0</Val>\n</Boolean>\n</Cluster>\n          <Cluster>\n            <Name>Alias</Name>\n            <NumElts>6</NumElts>\n            <String>\n              <Name>Name</Name>\n              <Val>Button_5</Val>\n</String>\n            <Array>\n              <Name>Route</Name>\n              <Dimsize>3</Dimsize>\n              <String>\n                <Name>String</Name>\n                <Val>M2H:2:1:1</Val>\n</String>\n              <String>\n                <Name>String</Name>\n                <Val>M2L:2:1:1</Val>\n</String>\n              <String>\n                <Name>String</Name>\n                <Val>M2L:2:16:1</Val>\n</String>\n</Array>\n            <Array>\n              <Name>UnRoute</Name>\n              <Dimsize>3</Dimsize>\n              <String>\n                <Name>String</Name>\n                <Val>M2H:2:1:0</Val>\n</String>\n              <String>\n                <Name>String</Name>\n                <Val>M2L:2:1:0</Val>\n</String>\n              <String>\n                <Name>String</Name>\n                <Val>M2L:2:16:1</Val>\n</String>\n</Array>\n            <String>\n              <Name>Description</Name>\n              <Val>Connect Button 5</Val>\n</String>\n            <String>\n              <Name>Group</Name>\n              <Val>Buttons</Val>\n</String>\n            <Boolean>\n              <Name>IsGroup</Name>\n              <Val>0</Val>\n</Boolean>\n</Cluster>\n          <Cluster>\n            <Name>Alias</Name>\n            <NumElts>6</NumElts>\n            <String>\n              <Name>Name</Name>\n              <Val>Button_6</Val>\n</String>\n            <Array>\n              <Name>Route</Name>\n              <Dimsize>3</Dimsize>\n              <String>\n                <Name>String</Name>\n                <Val>M2H:2:1:1</Val>\n</String>\n              <String>\n                <Name>String</Name>\n                <Val>M2L:2:1:1</Val>\n</String>\n              <String>\n                <Name>String</Name>\n                <Val>M2H:2:17:1</Val>\n</String>\n</Array>\n            <Array>\n              <Name>UnRoute</Name>\n              <Dimsize>3</Dimsize>\n              <String>\n                <Name>String</Name>\n                <Val>M2H:2:1:0</Val>\n</String>\n              <String>\n                <Name>String</Name>\n                <Val>M2L:2:1:0</Val>\n</String>\n              <String>\n                <Name>String</Name>\n                <Val>M2H:2:17:0</Val>\n</String>\n</Array>\n            <String>\n              <Name>Description</Name>\n              <Val>Connect Button 6</Val>\n</String>\n            <String>\n              <Name>Group</Name>\n              <Val>Buttons</Val>\n</String>\n            <Boolean>\n              <Name>IsGroup</Name>\n              <Val>0</Val>\n</Boolean>\n</Cluster>\n          <Cluster>\n            <Name>Alias</Name>\n            <NumElts>6</NumElts>\n            <String>\n              <Name>Name</Name>\n              <Val>RTC</Val>\n</String>\n            <Array>\n              <Name>Route</Name>\n              <Dimsize>0</Dimsize>\n              <String>\n                <Name>String</Name>\n                <Val/>\n</String>\n</Array>\n            <Array>\n              <Name>UnRoute</Name>\n              <Dimsize>0</Dimsize>\n              <String>\n                <Name>String</Name>\n                <Val/>\n</String>\n</Array>\n            <String>\n              <Name>Description</Name>\n              <Val>Real Time Clock</Val>\n</String>\n            <String>\n              <Name>Group</Name>\n              <Val>Active_Tests</Val>\n</String>\n            <Boolean>\n              <Name>IsGroup</Name>\n              <Val>1</Val>\n</Boolean>\n</Cluster>\n          <Cluster>\n            <Name>Alias</Name>\n            <NumElts>6</NumElts>\n            <String>\n              <Name>Name</Name>\n              <Val>Battery</Val>\n</String>\n            <Array>\n              <Name>Route</Name>\n              <Dimsize>4</Dimsize>\n              <String>\n                <Name>String</Name>\n                <Val>M2L:2:5:1</Val>\n</String>\n              <String>\n                <Name>String</Name>\n                <Val>M2L:2:27:1</Val>\n</String>\n              <String>\n                <Name>String</Name>\n                <Val>M2L:4:1:1</Val>\n</String>\n              <String>\n                <Name>String</Name>\n                <Val>M2L:4:28:1</Val>\n</String>\n</Array>\n            <Array>\n              <Name>UnRoute</Name>\n              <Dimsize>4</Dimsize>\n              <String>\n                <Name>String</Name>\n                <Val>M2L:2:5:0</Val>\n</String>\n              <String>\n                <Name>String</Name>\n                <Val>M2L:2:27:0</Val>\n</String>\n              <String>\n                <Name>String</Name>\n                <Val>M2L:4:1:0</Val>\n</String>\n              <String>\n                <Name>String</Name>\n                <Val>M2L:4:28:0</Val>\n</String>\n</Array>\n            <String>\n              <Name>Description</Name>\n              <Val>Connects PSU to battery holder</Val>\n</String>\n            <String>\n              <Name>Group</Name>\n              <Val>RTC</Val>\n</String>\n            <Boolean>\n              <Name>IsGroup</Name>\n              <Val>0</Val>\n</Boolean>\n</Cluster>\n</Array>\n        <Boolean>\n          <Name>Sim</Name>\n          <Val>1</Val>\n</Boolean>\n</Config>      <Ancestors>\n        <Ancestor>\n          <Class>SwitchBase</Class>\n          <Config>\n            <NumElts>1</NumElts>\n            <String>\n              <Name>default</Name>\n              <Val/>\n</String>\n</Config>        </Ancestor>\n      </Ancestors>\n    </Object>\n  </Objects>\n\n  <Ancestors>\n    <Ancestor>\n      <Class>SwitchBase</Class>\n      <Config>\n        <NumElts>1</NumElts>\n        <String>\n          <Name>default</Name>\n          <Val/>\n</String>\n</Config>    </Ancestor>\n  </Ancestors>\n\n</Object>\n"
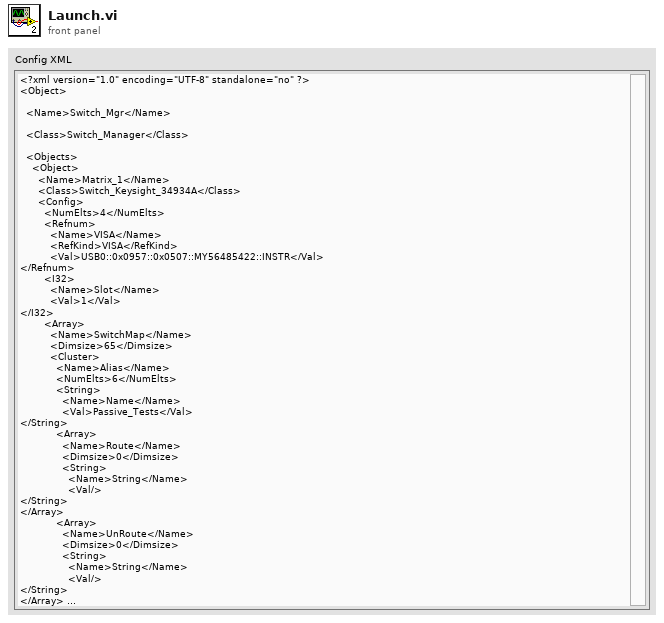
[diagram p1: front panel]
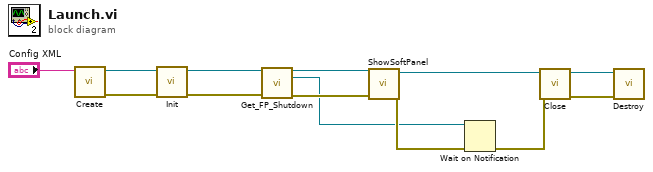
[diagram p0: block diagram]
diagram:
  n1 = call "Create.vi"("Config XML"="Config XML") -> ("error out"=w12:errorcluster, "reference out"=w13:refnum<class "ViPER.lvclass">)  [unwired: 9 in]
  n2 = call-dynamic "Init.vi"("error in (no error)"=w12, "reference in"=w13) -> ("error out"=w10:errorcluster, "reference out"=w11:refnum<class "ViPER.lvclass">)  [unwired: 8 in]
  n3 = call "Get_FP_Shutdown.vi"("ViPER_Base in"=w11, "error in (no error)"=w10) -> ("ViPER_Base out"=w9:refnum<class "ViPER.lvclass">, "SoftFP_Shutdown"=w6:refnum<notifier>, "error out"=w8:errorcluster)  [unwired: 9 in, 2 out]
  n4 = call-dynamic "ShowSoftPanel.vi"("error in (no error)"=w8, "Driver in"=w9) -> ("error out"=w7:errorcluster, "Driver out"=w5:refnum<class "ViPER.lvclass">)  [unwired: 7 in, 1 out]
  n5 = Wait on Notification(notifier=w6, error in (no error)=w7) -> (error out=w4:errorcluster)  [unwired: 2 in, 3 out]
  n6 = call-dynamic "Close.vi"("error in (no error)"=w4, "reference in"=w5) -> ("error out"=w3:errorcluster, "reference out"=w2:refnum<class "ViPER.lvclass">)  [unwired: 8 in]
  n7 = call "Destroy.vi"("error in (no error)"=w3, "reference in"=w2) -> ()  [unwired: 9 in, 1 out]
